vi "累积剂量查询模块.vi"() -> ()   [LabVIEW 2017]
uses:
  <vilib>/Utility/miscctls.llb/LVRowAndColumnTypeDef.ctl
  <vilib>/Utility/miscctls.llb/LVRowAndColumnUnsignedTypeDef.ctl
panel:
  in  "计数标志-刷新":i32
  in  "定时器":T1
  out "定时触发VI-引用":refnum<vi>
  in  "设备列表":T2[](array[typedef])
  in  "探测器列表":i32(listbox)
  in  "自定义导出":bool
  in  "导出条件":T5
  in  "XY图赋值错误":errorcluster caption="错误输出"
  out "刷新数据库错误":errorcluster caption="error out"
  in  "查看导出":bool
  in  "菜单项-报警列表":T6
  in  "菜单项-累积列表":T7
  in  "报警单元格位置":T8 caption="单元格位置"
  in  "累积单元格位置":T8 caption="单元格位置"
  out "信号-停止":bool=TRUE
  out "信号-刷新":bool=TRUE
  in  "刷新":bool
  in  "列数-累积表":u32
  in  "列数-报警表":u32
  out "错误输出":errorcluster
  out "累积列表选中索引":i32
  out "报警列表选中索引":i32
  out "事件-报警列表选中":refnum<user-event>
  out "事件-累积列表选中":refnum<user-event>
  in  "探测器的绑定数据":T13(array[cluster])
  out "累积剂量记录":i32(listbox)
  out "报警记录":i32(listbox)
  in  "XY图":cluster{"时间":timestamp[], "测量值":dbl[]}[](graph)
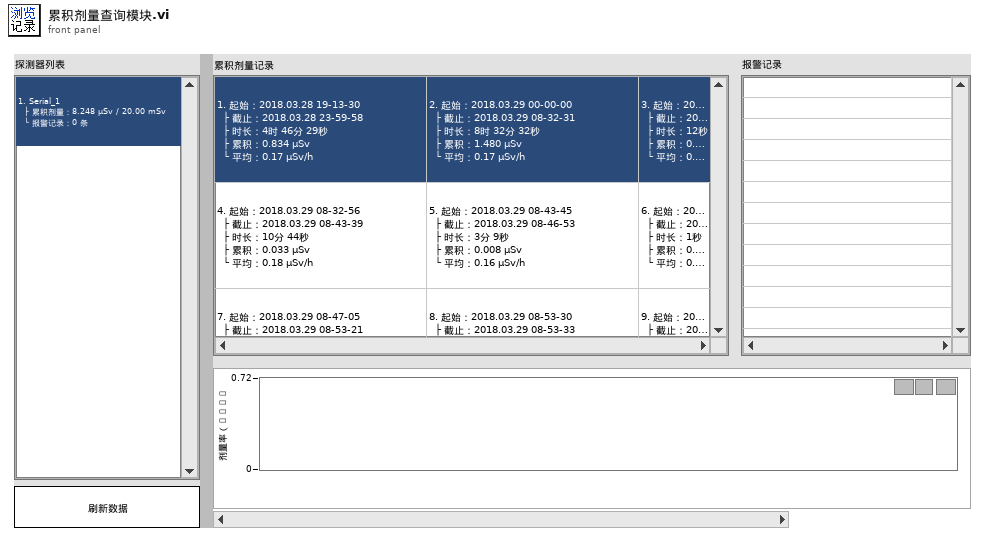
[diagram p1: front panel]
types:
  T1 = typedef "定时器枚举.ctl" = enum16{"累积定时", "导出定时"}
  T2 = typedef "探测器信息.ctl" = cluster{"网络地址":string, "名称":string, "备注":string, "累积剂量":dbl, "累积限值":dbl, "硬件剂量率限值":T3, "剂量率限值1":dbl, "剂量率限值2":dbl, "报警方式":T4}
  T3 = typedef "探头剂量率限值选择.ctl" = enum16{"一级限值", "二级限值"}
  T4 = typedef "报警方式选择.ctl" = enum16{"常报警", "自动静音", "手动静音"}
  T5 = typedef "文件导出条件.ctl" = cluster{"起始(包含)":timestamp, "截止(不含)":timestamp, "分别导出?":bool}
  T6 = typedef "菜单项-浏览界面-报警列表.ctl" = enum16{"预览"}
  T7 = typedef "菜单项-浏览界面-累积列表.ctl" = enum16{"删除选中时段"}
  T8 = typedef "LVRowAndColumnTypeDef.ctl" = cluster{"Row":i32, "Column":i32}
  T9 = typedef "单条累积记录.ctl" = cluster{"起始时间":timestamp, "结束时间":timestamp, "累积剂量":dbl}
  T10 = typedef "通用报警记录.ctl" = cluster{"探头状态":T11, "探头地址与信息":T2, "缓存绘图数据":T12, "平均值":dbl, "报警时长":cluster{"分":u16, "秒":u16}, "结论":string}
  T11 = typedef "探头状态.ctl" = enum16{"正常", "离线", "禁用", "一级报警", "二级报警", "累积报警"}
  T12 = typedef "时值缓存压缩模块.lvlib/缓存数据.ctl" = cluster{"时间":timestamp[], "数值":dbl[], "压缩等级数量":i32[], "最大值":cluster{"时间":timestamp, "数值":dbl}, "起始点":cluster{"时间":timestamp, "数值":dbl}, "容量限值":i32, "报警累积":dbl}
  T13 = cluster{"累积曲线数据":T9[], "累积列表内容":string[], "匹配的报警数据":cluster{"名称":string, "路径":path, "内容":string, "报警记录":T10}[]}[]
  T14 = typedef "浏览XY图曲线索引.ctl" = enum16{"最大值-选中", "最大值点", "率警-选中", "率警", "累积-选中", "累积-超限", "累积"}
  T15 = typedef "簇-输入.ctl" = cluster{"配置文件动作":T16, "数据输入":variant}
  T16 = typedef "枚举-配置文件动作.ctl" = enum16{"初始化加载配置", "读取配置", "写入-屏幕键盘", "写入-静音延迟", "写入-主要探头类型", "写入-串口配置", "写入-累积定时", "写入-导出定时", "保存配置到文件"}
  T17 = enum32{"Invalid", "Standard", "Closed", "Hidden", "Minimized", "Maximized"}
  T18 = typedef "簇-定时配置.ctl" = cluster{"定时模式":enum16{"绝对时间", "相对时间"}, "单位":enum16{"年", "月", "日", "时", "分"}, "间隔":u8, "目标时刻":timestamp}
  T19 = typedef "删除记录输入.ctl" = cluster{"名称":string, "多条记录(空则全删)":T9[]}
  T20 = typedef "DB动作与数据.ctl" = cluster{"动作类型":T21, "输入数据":variant}
  T21 = typedef "DB动作类型.ctl" = enum16{"DB-文件初始化+连接", "DB-断开连接", "DB-结构初始化", "DB-加载设备", "DB-检查连接状态", "设备-登记新设备+数据表", "设备-删除设备", "设备-修改网址", "设备-修改名称+转移数据", "设备-修改备注", "设备-修改限值", "设备-累积校准", "设备-重排", "数据-获取全部", "数据-删除数据", "数据-写改累积记录+改累积剂量", "读变量-全部设备"}
  T22 = typedef "簇-配置文件内容.ctl" = cluster{"调试模式？":bool, "屏幕键盘？":bool, "软件版本":string, "静音延迟 s":u16, "主要探头类型":T23, "串口配置":cluster{"COM口":refnum<visa-resource-name>, "波特率":enum16{"9600", "19200"}, "读写超时ms":i16, "丢包判定次数":i16}, "定时配置-累积分段":T18, "定时配置-自动导出":cluster{"定时配置-自动导出":T18, "分别导出?":bool}}
  T23 = typedef "枚举-主要探头类型.ctl" = enum16{"网络探头", "串口探头"}
  T24 = typedef "LVRowAndColumnUnsignedTypeDef.ctl" = cluster{"Row":u32, "Column":u32}
  T25 = cluster{"累积曲线数据":T9[], "累积列表内容":string[], "匹配的报警数据":cluster{"名称":string, "路径":path, "内容":string, "报警记录":T10}[]}
  T26 = cluster{"Shift":bool, "Ctrl":bool, "Alt":bool, "Cmd":bool, "Opt":bool}
  T27 = typedef "LVPoint32TypeDef.ctl" = cluster{"Horizontal":i32, "Vertical":i32}
  T28 = typedef "改动项选择.ctl" = enum16{"未改动", "改动-启用状态", "改动-探头信息", "改动-报警限值", "动作-手动静音", "动作-重启累积时段", "动作-累积删除", "动作-重连"}
  T29 = typedef "改动项.ctl" = cluster{"改动项选择":T28, "启用？":bool, "探测器信息":T2}
  T30 = typedef "探头属性.ctl" = cluster{"探头地址与信息":T2, "测量值":T31, "限值":T32, "探头状态":T11, "累积记录":T9, "报警方式":T33}
  T31 = typedef "测量值.ctl" = cluster{"时间":timestamp, "数值":dbl}
  T32 = typedef "剂量率限值.ctl" = cluster{"限值1":dbl, "限值2":dbl, "探头限值":T3}
  T33 = typedef "报警方式.ctl" = cluster{"报警方式":T4, "延迟计时":u16, "报警中？":bool}
  T34 = cluster{"名称":string, "路径":path, "内容":string, "报警记录":T10}[]
  T35 = cluster{"名称":string, "路径":path, "内容":string, "报警记录":T10}
  T36 = typedef "LVRectTypeDef.ctl" = cluster{"Left":i16, "Top":i16, "Right":i16, "Bottom":i16}
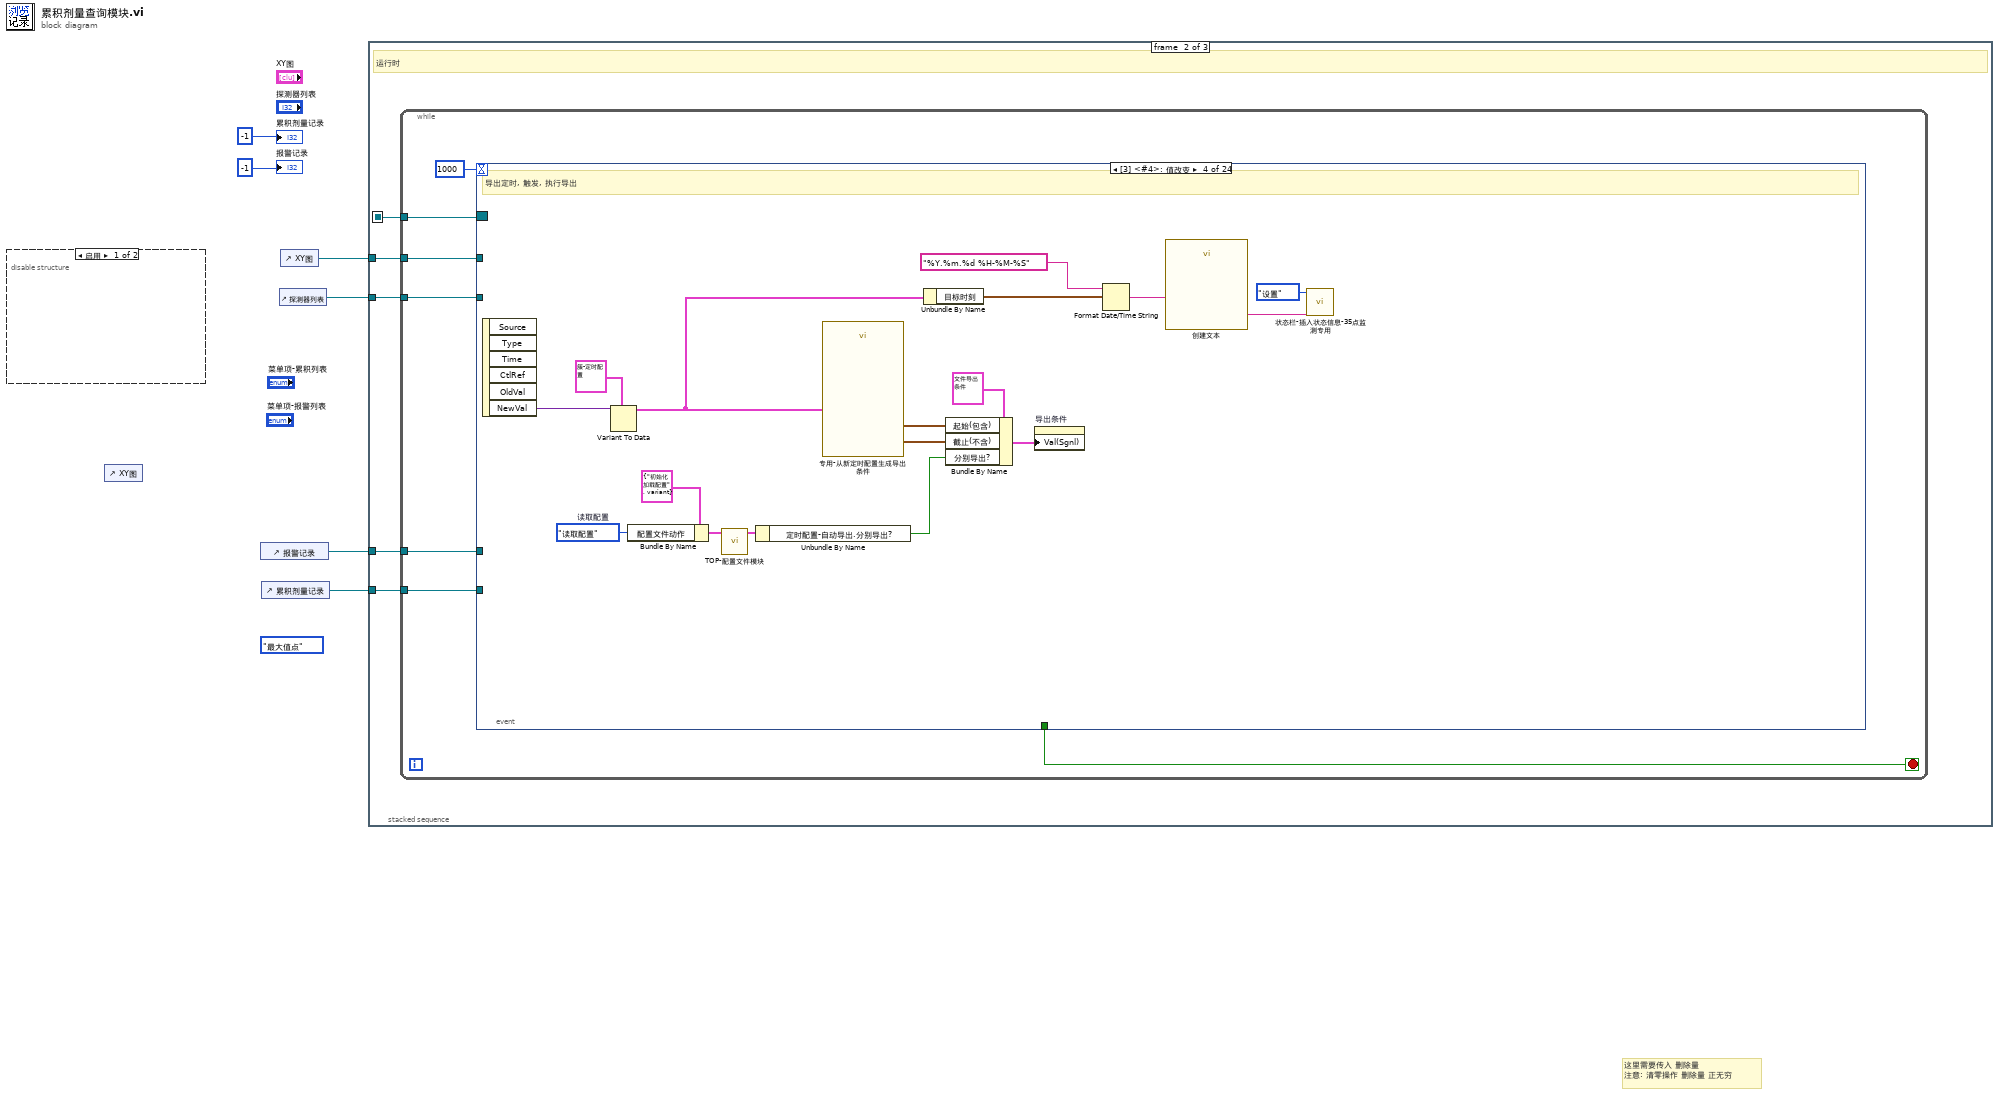
[diagram p0: block diagram]
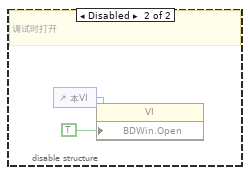
[diagram p2: hidden frame]
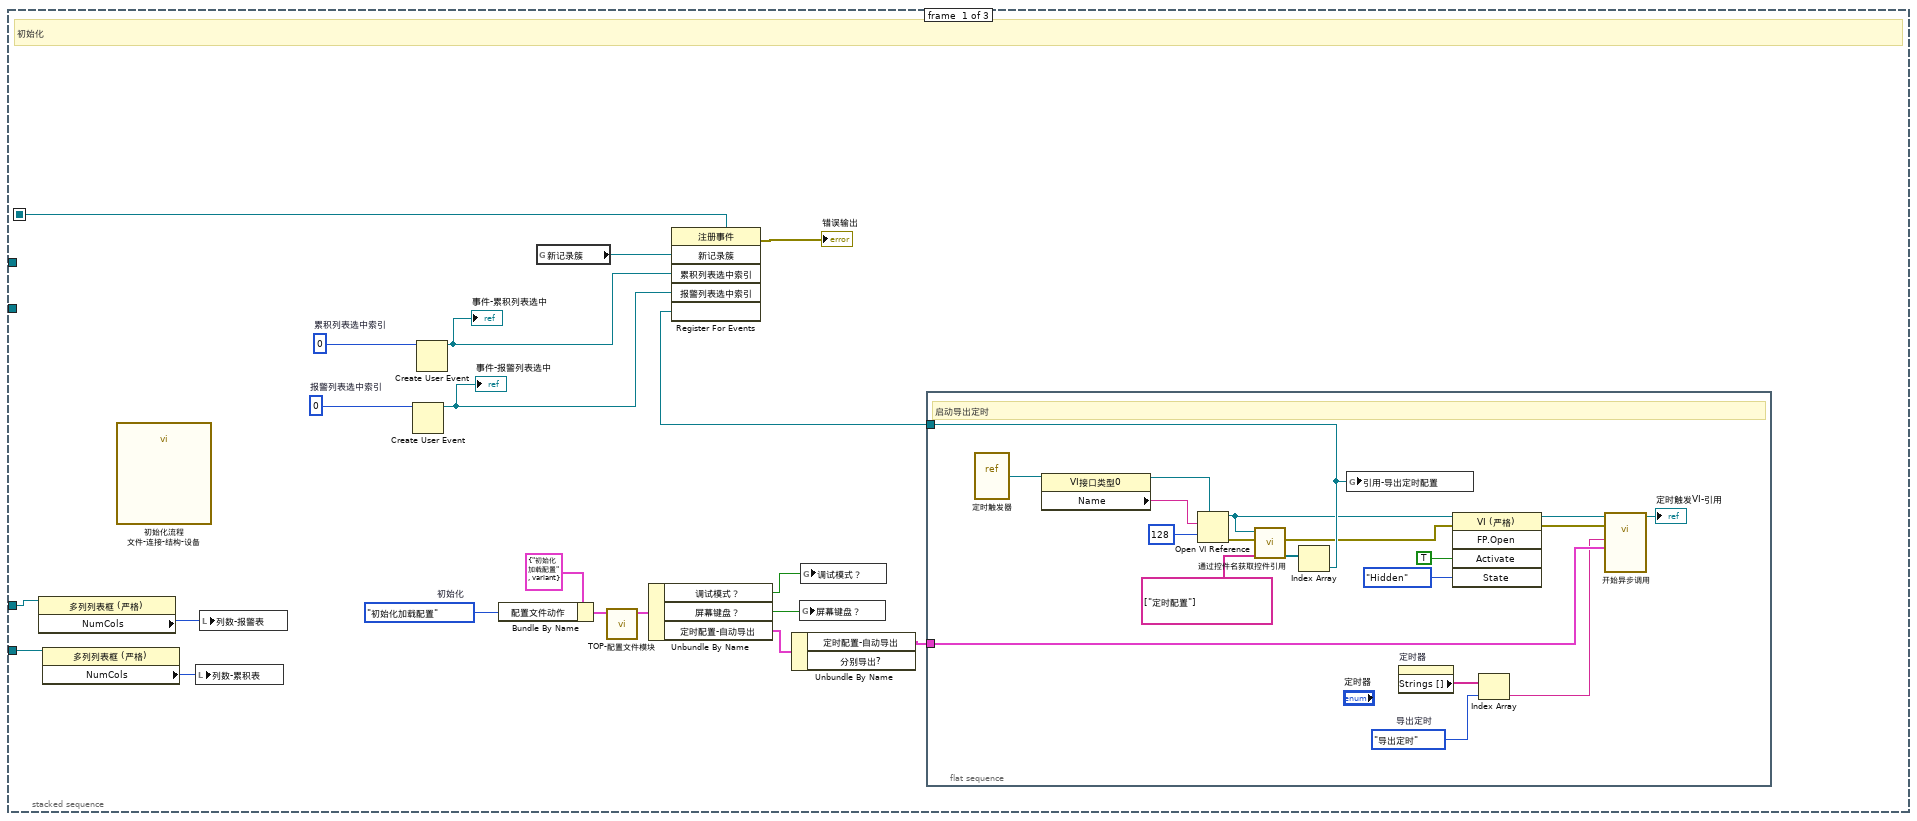
[diagram p3: hidden frame]
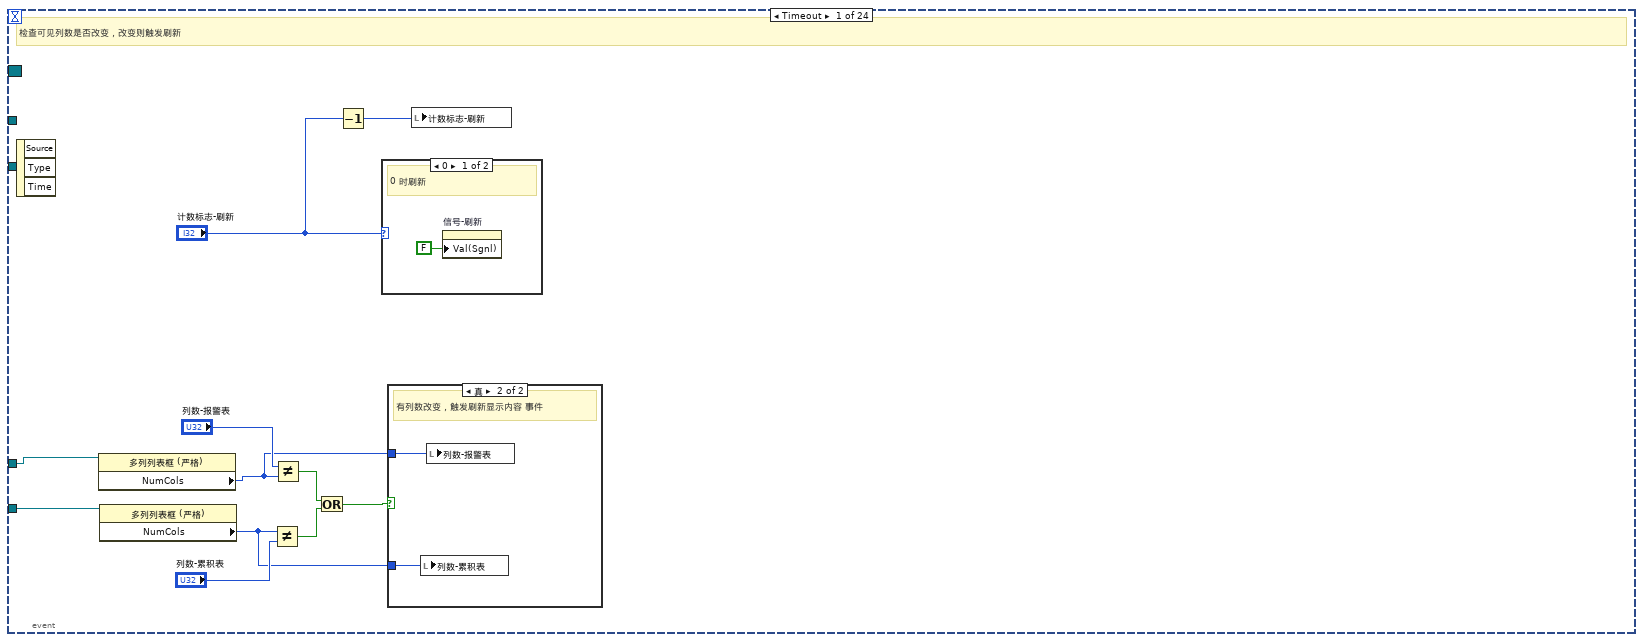
[diagram p4: hidden frame]
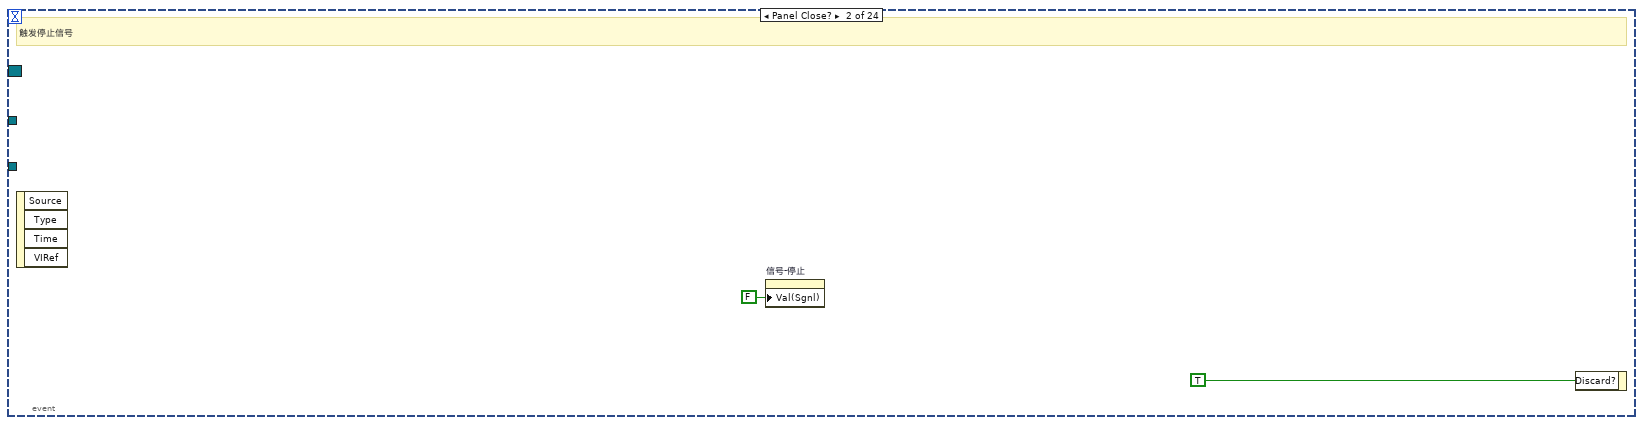
[diagram p7: hidden frame]
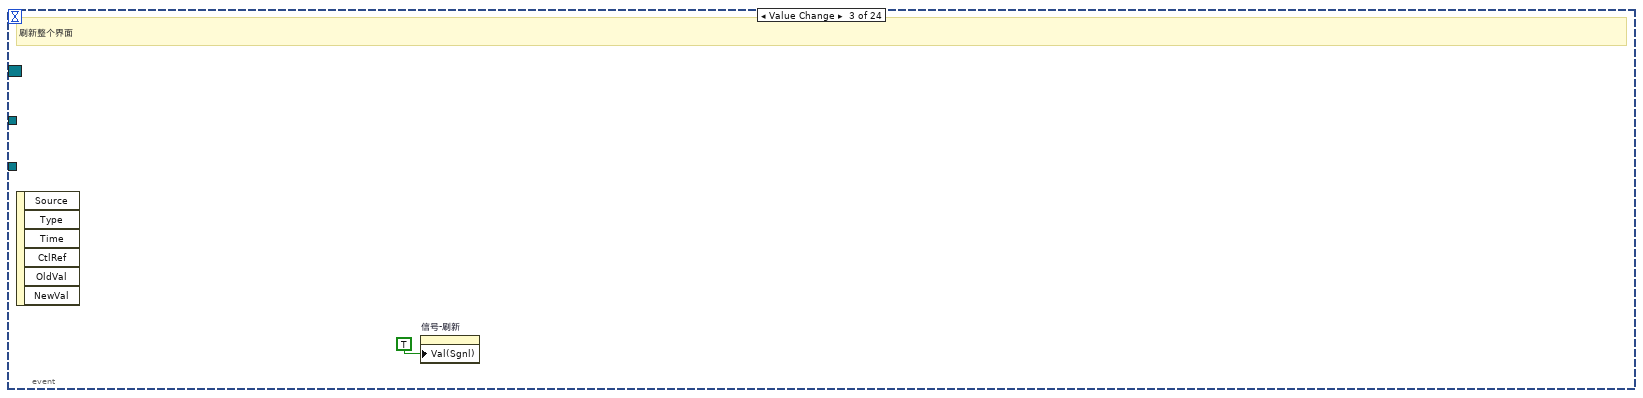
[diagram p8: hidden frame]
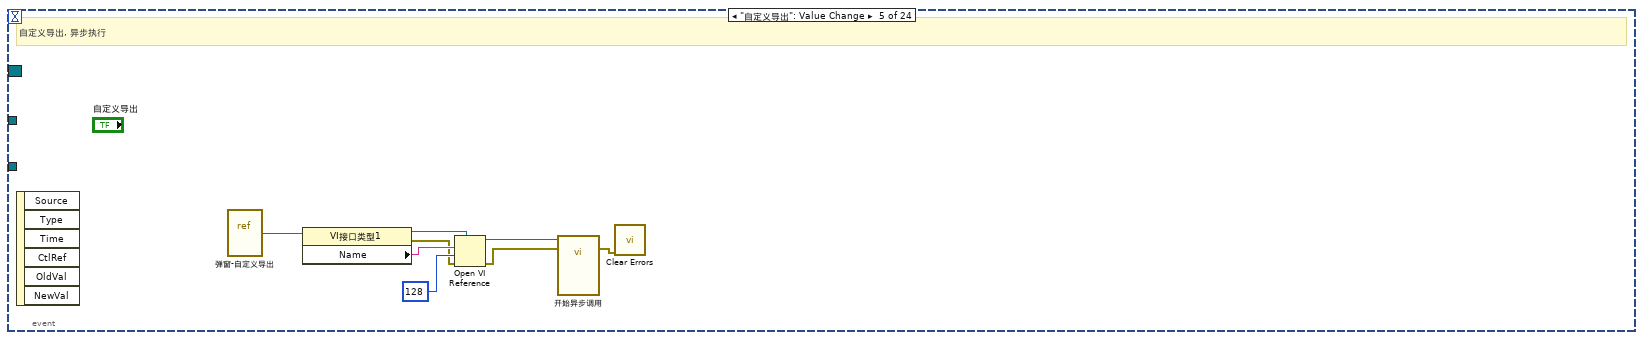
[diagram p9: hidden frame]
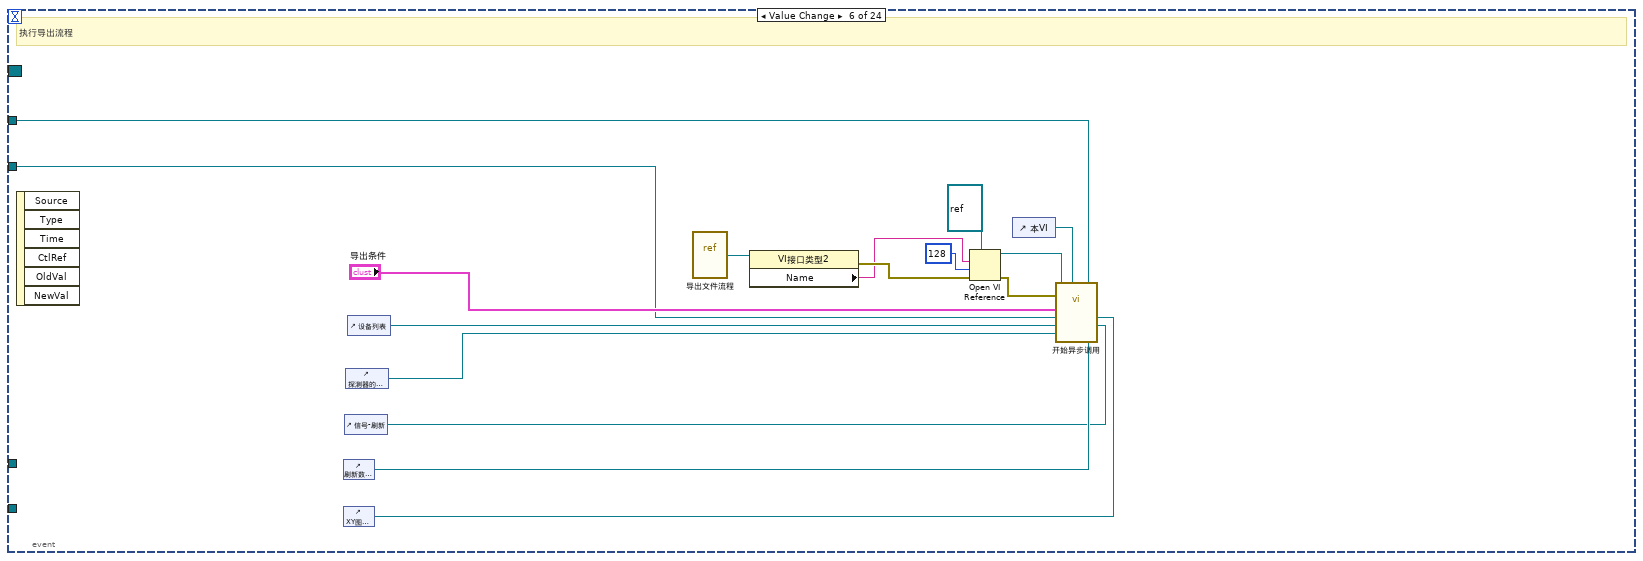
[diagram p10: hidden frame]
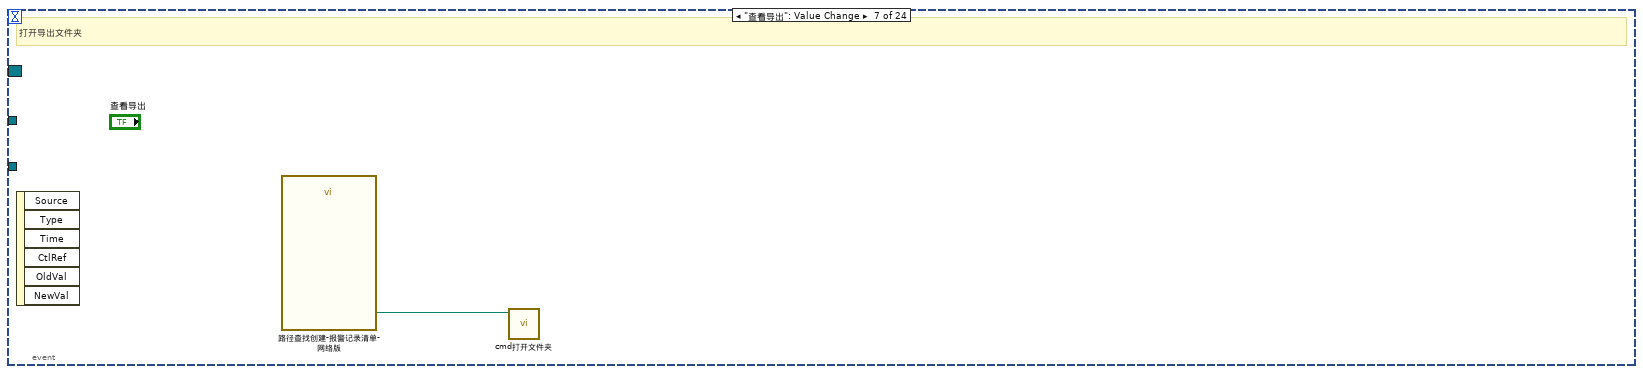
[diagram p11: hidden frame]
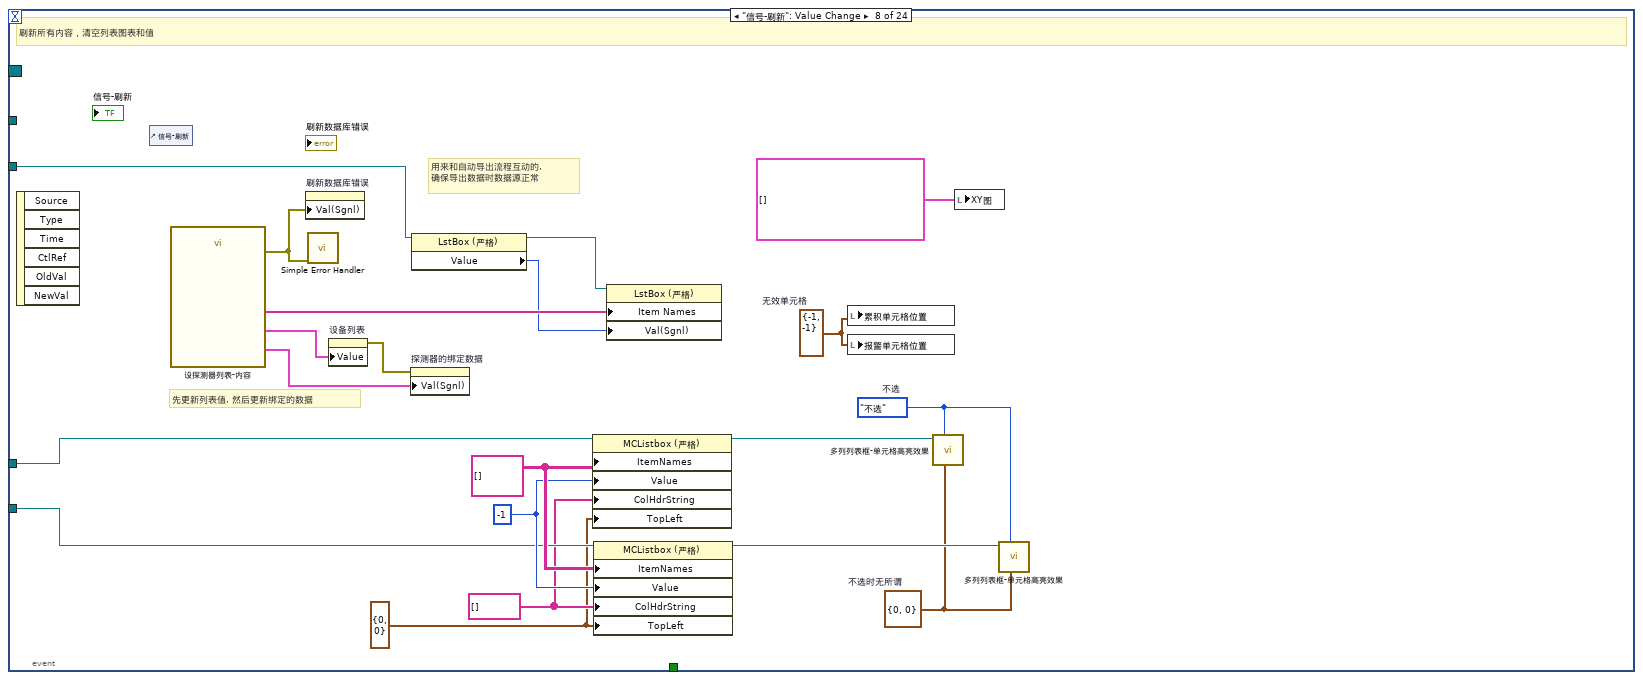
[diagram p12: hidden frame]
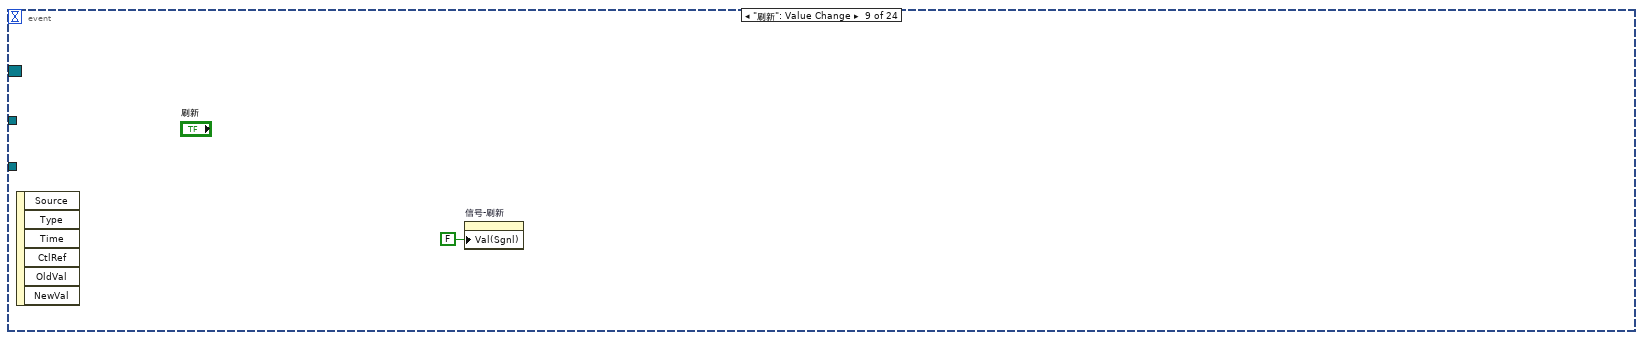
[diagram p13: hidden frame]
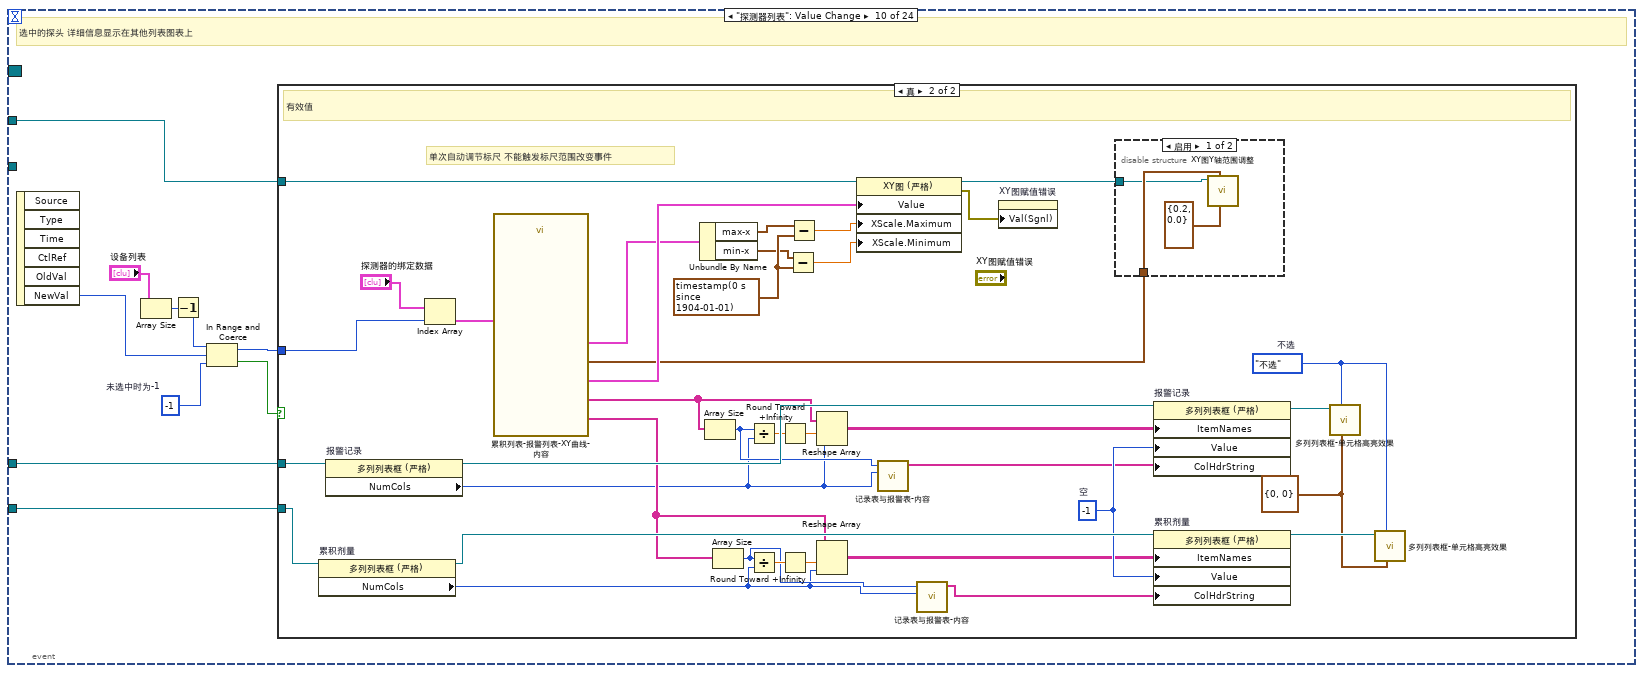
[diagram p14: hidden frame]
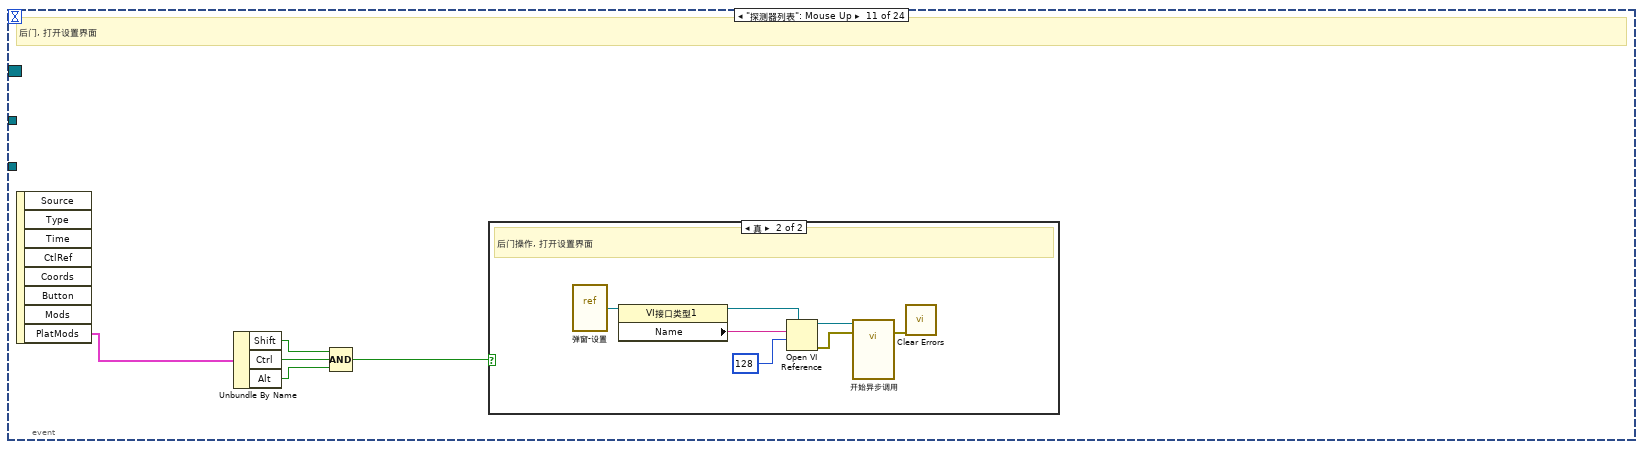
[diagram p17: hidden frame]
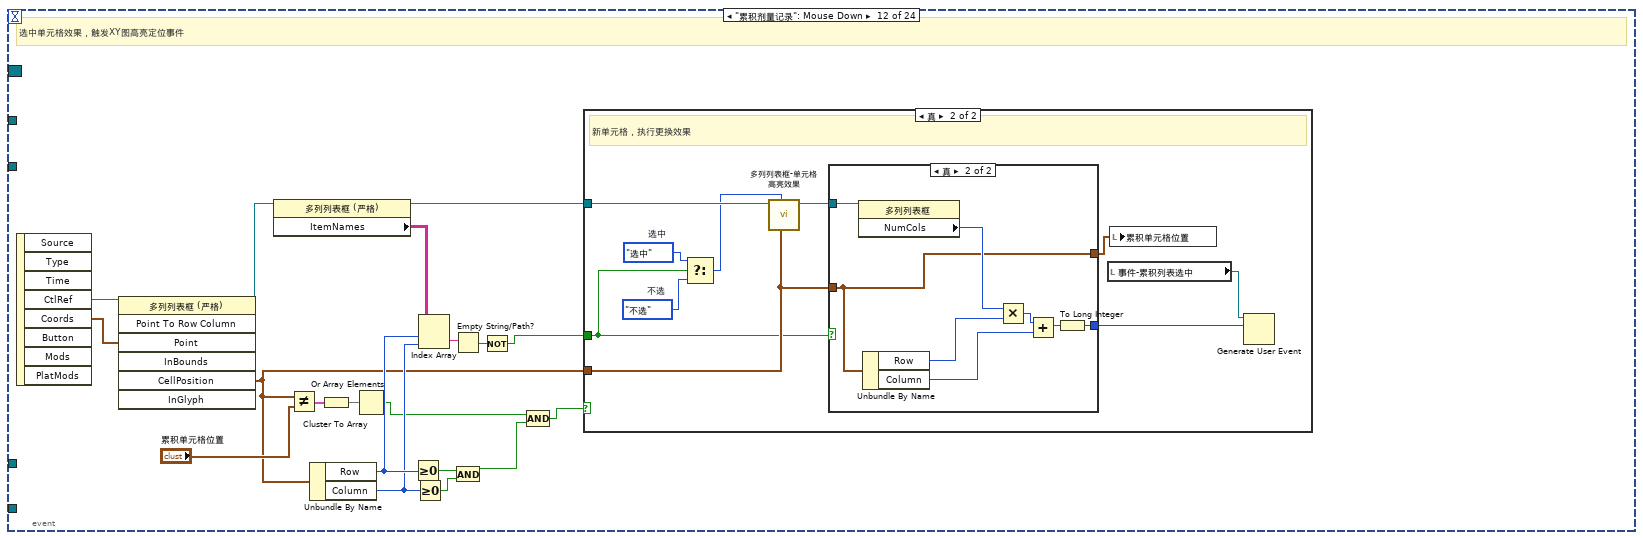
[diagram p19: hidden frame]
diagram:
  (unwired) 浏览XY图曲线索引."最大值点"
  # "这里需要传入 删除量\n注意: 清零操作 删除量 正无穷"
  n1 = disable-structure shown="启用" {
    frame Enabled {
    }
    frame Disabled {
      # "调试时打开"
      n2 = control-ref of="本VI"() -> (w7:refnum<vi>)
      n3 = property class="VI"(reference=w7, "BDWin.Open"=TRUE ("程序框图窗口:打开")) -> ()  [unwired: 1 in, 2 out]
    }
  }
  n4 = control-ref of="XY图"() -> ()  [unwired: 1 out]
  n5 = control-ref of="报警记录"() -> (w5:refnum<vi>)
  n6 = control-ref of="累积剂量记录"() -> (w4:refnum<vi>)
  n7 = control-ref of="探测器列表"() -> (w6:refnum<vi>)
  n8 = control-ref of="XY图"() -> (w3:refnum<vi>)
  n9 = stacked-sequence {
    seq-local: [w27 _ _] -> [_ w52 _]
    tunnel: w6 -> [_ w51 _]
    tunnel: w5 -> [w21 w50 _]
    tunnel: w4 -> [w20 w49 _]
    tunnel: w3 -> [_ w48 _]
    frame #0 {
      w16 = 枚举-配置文件动作."初始化加载配置"  # 初始化
      w24 = 0  # 报警列表选中索引
      w26 = 0  # 累积列表选中索引
      # "初始化"
      n10 = property class="多列列表框 (严格)"(reference=w21) -> ("NumCols"=w19:u32)  [unwired: 1 in, 2 out]
      n11 = property class="多列列表框 (严格)"(reference=w20) -> ("NumCols"=w18:u32)  [unwired: 1 in, 2 out]
      n12 = call "初始化流程 文件-连接-结构-设备.vi"() -> ()  [unwired: 10 in, 2 out]
      n13 = local write "列数-累积表"(w18) -> ()
      n14 = local write "列数-报警表"(w19) -> ()
      n15 = Create User Event(user event datatype=w24) -> (user event=w23:refnum<user-event>)  [unwired: 1 in, 1 out]
      "事件-报警列表选中" <- w23
      n16 = Create User Event(user event datatype=w26) -> (user event=w25:refnum<user-event>)  [unwired: 1 in, 1 out]
      "事件-累积列表选中" <- w25
      n17 = Bundle By Name(cluster=T15 {"配置文件动作"=enum."初始化加载配置", "数据输入"=variant} ("输入"), "配置文件动作"=w16) -> (w13:T15)
      n18 = global read "全局变量-35点监测.vi" "新记录簇"() -> (w28:refnum<vi>)
      n19 = call "TOP-配置文件模块.vi"("输入"=w13) -> ("配置文件"=w14:T22)  [unwired: 9 in, 1 out]
      n20 = Unbundle By Name(w14) -> ("调试模式？"=w10:bool, "屏幕键盘？"=w9:bool, "定时配置-自动导出"=w12:cluster{"定时配置-自动导出":T18, "分别导出?":bool})
      n21 = register-events(w28, w25, w23, w17) -> (reference out=w27:refnum<event-registration>, error out=→"错误输出":errorcluster)  [unwired: 2 in]
      n22 = Unbundle By Name(w12) -> ("定时配置-自动导出"=w11:T18)  [unwired: 1 out]
      n23 = global write "全局变量-35点监测.vi" "屏幕键盘？"(w9) -> ()
      n24 = global write "全局变量-35点监测.vi" "调试模式？"(w10) -> ()
      n25 = flat-sequence {
        tunnel: w11 -> [w40]
        tunnel: [w41] -> w17
        frame #0 {
          w31 = 定时器枚举."导出定时"  # 导出定时
          # "启动导出定时"
          n26 = vi-ref "定时触发器.vi"() -> (w45:refnum<vi>)
          n27 = property class="VI接口类型0"(reference=w45) -> (reference out=w29:refnum<vi>, "Name"=w47:string)  [unwired: 1 in, 1 out]
          n28 = Open VI Reference(type specifier VI Refnum (for type only)=w29, vi path=w47, options=128 ("选项")) -> (vi reference=w39:refnum<vi>, error out=w36:errorcluster)  [unwired: 3 in]
          n29 = call "通过控件名获取控件引用.vi"("控件名数组"=string[] ["定时配置"], "错误输入（无错误）"=w36, "VI引用"=w39) -> ("控件引用输出"=w43:refnum<vi>[], "错误输出"=w37:errorcluster)  [unwired: 6 in, 1 out]
          n30 = Index Array(array=w43) -> (element=w41:refnum<vi>)  [unwired: 1 in]
          n31 = global write "全局变量-35点监测.vi" "引用-导出定时配置"(w41) -> ()
          n32 = property on="定时器" class="Enum (严格)"() -> ("Strings []"=w32:string[])  [unwired: 2 in, 2 out]
          n33 = invoke class="VI (严格)" method="FP.Open"(reference=w39, error in=w37, "Activate"=TRUE ("激活？"), "State"=T17."Hidden" ("状态")) -> (reference out=w38:refnum<vi>, error out=w35:errorcluster)  [unwired: 1 in, 3 out]
          n34 = Index Array(array=w32, index=w31) -> (element=w30:string)
          n35 = call-by-ref "开始异步调用"(reference=w38, error in=w35, "定时配置"=w40, "定时器结构名"=w30) -> (reference out=→"定时触发VI-引用":refnum<vi>)  [unwired: 10 in, 1 out]
        }
      }
    }
    frame #1 {
      # "运行时"
      n36 = while {
        tunnel: w52 -> [w58]
        tunnel: w51 -> [w57]
        tunnel: w50 -> [w56]
        tunnel: w49 -> [w55]
        tunnel: w48 -> [w54]
        stop <- w59 stop-if-true
        n37 = event shown="[3] <#4>: 值改变" {
          selector: w58 -> [_ _ _ _ _ _ _ _ _ _ _ _ _ _ _ _ _ _ _ _ _ _ _ w578]
          dyn-events: _ -> [_ _ _ _ _ _ _ _ _ _ _ _ _ _ _ _ _ _ _ _ _ _ _ _]
          timeout: 1000 -> [_ _ _ _ _ _ _ _ _ _ _ _ _ _ _ _ _ _ _ _ _ _ _ _]
          tunnel: [_ _ _ _ _ _ _ _ _ _ _ _ _ _ _ _ _ _ _ _ _ _ _ TRUE ("放弃？")] -> w59
          tunnel: w57 -> [_ _ _ _ _ w116 _ w127 _ _ _ _ _ _ _ _ _ _ _ _ _ _ _ _]
          tunnel: w56 -> [w70 _ _ _ _ _ _ w137 _ w142 _ _ _ _ _ _ _ _ _ _ _ w443 _ _]
          tunnel: w55 -> [w69 _ _ _ _ _ _ w134 _ w143 _ _ _ _ _ _ _ _ _ _ _ w442 _ _]
          tunnel: w54 -> [_ _ _ _ _ w110 _ _ _ w141 _ _ _ _ _ _ w323 w342 _ _ _ _ _ _]
          event Timeout {
            # "检查可见列数是否改变，改变则触发刷新"
            n38 = event-data() -> ()  [unwired: 1 in, 3 out]
            n39 = property class="多列列表框 (严格)"(reference=w70) -> ("NumCols"=w62:u32)  [unwired: 1 in, 2 out]
            n40 = property class="多列列表框 (严格)"(reference=w69) -> ("NumCols"=w63:u32)  [unwired: 1 in, 2 out]
            n41 = Not Equal?(x=w63, y="列数-累积表") -> (x != y?=w66:bool)
            n42 = Not Equal?(x="列数-报警表", y=w62) -> (x != y?=w65:bool)
            n43 = Or(x=w65, y=w66) -> (x .or. y?=w64:bool)
            n44 = Decrement(x="计数标志-刷新") -> (x-1=w60:i32)
            n45 = case shown="0" "计数标志-刷新" {
              frame 0 {
                # "0 时刷新"
                n46 = property on="信号-刷新" class="Bool (严格)"("Val(Sgnl)"=FALSE ("值(信号)")) -> ()  [unwired: 2 in, 2 out]
              }
              frame 1, Default {
              }
            }
            n47 = case shown="真" w64 {
              tunnel: w63 -> [_ w72]
              tunnel: w62 -> [_ w73]
              frame False {
              }
              frame True {
                # "有列数改变，触发刷新显示内容 事件"
                n48 = local write "列数-累积表"(w72) -> ()
                n49 = local write "列数-报警表"(w73) -> ()
              }
            }
            n50 = local write "计数标志-刷新"(w60) -> ()
          }
          event Panel Close? {
            # "触发停止信号"
            n51 = event-data() -> ()  [unwired: 1 in, 4 out]
            n52 = property on="信号-停止" class="Bool (严格)"("Val(Sgnl)"=FALSE ("值(信号)")) -> ()  [unwired: 2 in, 2 out]
            n53 = event-data("Discard?"=TRUE ("放弃？")) -> ()  [unwired: 1 in, 1 out]
          }
          event Value Change {
            # "刷新整个界面"
            n54 = event-data() -> ()  [unwired: 1 in, 6 out]
            n55 = property on="信号-刷新" class="Bool (严格)"("Val(Sgnl)"=TRUE ("值(信号)")) -> ()  [unwired: 2 in, 2 out]
          }
          event Value Change {
            w85 = 枚举-配置文件动作."读取配置"  # 读取配置
            # "导出定时, 触发, 执行导出"
            n56 = event-data() -> ("NewVal"=w93:variant)  [unwired: 1 in, 5 out]
            n57 = Variant To Data(type=T18 {"定时模式"=enum."绝对时间", "单位"=enum."年", "间隔"=1, "目标时刻"=timestamp(0 s since 1904-01-01)} ("定时配置"), Variant=w93) -> (data=w82:T18)  [unwired: 1 in, 1 out]
            n58 = Bundle By Name(cluster=T15 {"配置文件动作"=enum."初始化加载配置", "数据输入"=variant} ("输入"), "配置文件动作"=w85) -> (w86:T15)
            n59 = call "TOP-配置文件模块.vi"("输入"=w86) -> ("配置文件"=w84:T22)  [unwired: 9 in, 1 out]
            n60 = Unbundle By Name(w84) -> ("定时配置-自动导出.分别导出?"=w83:bool)
            n61 = call "专用-从新定时配置生成导出条件.vi"("定时配置"=w82) -> ("时间上限(不含)"=w89:timestamp, "时间下限(包含)"=w90:timestamp)  [unwired: 9 in]
            n62 = Unbundle By Name(w82) -> ("目标时刻"=w80:timestamp)
            n63 = Bundle By Name(cluster=T5 {"起始(包含)"=timestamp(0 s since 1904-01-01), "截止(不含)"=timestamp(0 s since 1904-01-01), "分别导出?"=FALSE} ("导出条件"), "起始(包含)"=w90, "截止(不含)"=w89, "分别导出?"=w83) -> (w88:T5)
            n64 = property on="导出条件" class="Clust (严格)"("Val(Sgnl)"=w88) -> ()  [unwired: 2 in, 2 out]
            n65 = Format Date/Time String(time format string (%c)="%Y.%m.%d %H-%M-%S" ("时间格式字符串(%c)"), seconds (now)=w80) -> (date/time string=w78:string)  [unwired: 1 in]
            n66 = call "创建文本"("下个_导时"=w78) -> ("Result"=w77:string)  [unwired: 13 in, 1 out]
            n67 = call "状态栏-插入状态信息-35点监测专用.vi"("消息内容"=w77, "状态类型"=enum16{"全部", "报警", "通信", "设置"}."设置") -> ()  [unwired: 10 in]
          }
          event "自定义导出": Value Change {
            # "自定义导出, 异步执行"
            n68 = event-data() -> ()  [unwired: 1 in, 6 out]
            n69 = vi-ref "弹窗-自定义导出.vi"() -> (w101:refnum<vi>)
            n70 = property class="VI接口类型1"(reference=w101) -> (reference out=w94:refnum<vi>, error out=w97:errorcluster, "Name"=w100:string)  [unwired: 1 in]
            n71 = Open VI Reference(type specifier VI Refnum (for type only)=w94, vi path=w100, options=128 ("选项"), error in (no error)=w97) -> (vi reference=w99:refnum<vi>, error out=w96:errorcluster)  [unwired: 2 in]
            n72 = call-by-ref "开始异步调用"(reference=w99, error in=w96) -> (error out=w95:errorcluster)  [unwired: 12 in, 1 out]
            n73 = call <vilib>:"Clear Errors.vi"("error in (no error)"=w95) -> ()  [unwired: 5 in, 2 out]
          }
          event Value Change {
            # "执行导出流程"
            n74 = event-data() -> ()  [unwired: 1 in, 6 out]
            n75 = control-ref of="刷新数据库错误"() -> (w113:refnum<vi>)
            n76 = control-ref of="XY图赋值错误"() -> (w111:refnum<vi>)
            n77 = control-ref of="信号-刷新"() -> (w112:refnum<vi>)
            n78 = control-ref of="探测器的绑定数据"() -> (w114:refnum<vi>)
            n79 = control-ref of="设备列表"() -> (w115:refnum<vi>)
            n80 = vi-ref "导出文件流程.vi"() -> (w109:refnum<vi>)
            n81 = property class="VI接口类型2"(reference=w109) -> (error out=w108:errorcluster, "Name"=w107:string)  [unwired: 1 in, 1 out]
            n82 = Open VI Reference(type specifier VI Refnum (for type only)=refnum<vi> refnum ("类型说明符VI引用句柄（仅用于类型）"), vi path=w107, options=128 ("选项"), error in (no error)=w108) -> (vi reference=w104:refnum<vi>, error out=w103:errorcluster)  [unwired: 2 in]
            n83 = control-ref of="本VI"() -> (w102:refnum<vi>)
            n84 = call-by-ref "开始异步调用"(reference=w104, error in=w103, "刷新错误?"=w113, "刷新信号-引用"=w112, "XY图更新错误?"=w111, "XY图-引用"=w110, "查询界面VI-引用"=w102, "累积记录-引用"=w114, "设备清单-引用"=w115, "设备列表-引用"=w116, "导出条件"="导出条件") -> ()  [unwired: 2 in, 3 out]
          }
          event "查看导出": Value Change {
            # "打开导出文件夹"
            n85 = event-data() -> ()  [unwired: 1 in, 6 out]
            n86 = call "路径查找创建-报警记录清单-网络版.vi"() -> ("导出记录"=w118:path)  [unwired: 2 in, 13 out]
            n87 = call "cmd打开文件夹.vi"("文件路径"=w118) -> ()  [unwired: 10 in, 1 out]
          }
          event "信号-刷新": Value Change {
            w119 = T24 {"Row"=0, "Column"=0} ("左上可见单元格")
            w124 = string[] [] ("项名")
            w128 = enum16{"选中", "不选"}."不选"  # 不选
            w129 = T8 {"Row"=0, "Column"=0}  # 不选时无所谓
            w130 = T8 {"Row"=-1, "Column"=-1}  # 无效单元格
            w135 = -1 ("值")
            w136 = string[][] [] ("项名")
            # "用来和自动导出流程互动的,\n确保导出数据时数据源正常"
            # "先更新列表值, 然后更新绑定的数据"
            # "刷新所有内容，清空列表图表和值"
            n88 = event-data() -> ()  [unwired: 1 in, 6 out]
            n89 = control-ref of="信号-刷新"() -> ()  [unwired: 1 out]
            n90 = call "设探测器列表-内容.vi"() -> ("error out"=w120:errorcluster, "探测器的绑定数据"=w122:T13, "探测器列表内容"=w138:string[], "设备列表"=w123:T2[])  [unwired: 8 in]
            n91 = property on="刷新数据库错误" class="Clust (严格)"("Val(Sgnl)"=w120) -> ()  [unwired: 2 in, 2 out]
            n92 = call <vilib>:"Simple Error Handler.vi"("error in (no error)"=w120) -> ()  [unwired: 4 in, 5 out]
            n93 = property on="设备列表" class="Arr (严格)"("Value"=w123) -> (error out=w121:errorcluster)  [unwired: 2 in, 1 out]
            n94 = property on="探测器的绑定数据" class="Arr (严格)"(error in=w121, "Val(Sgnl)"=w122) -> ()  [unwired: 1 in, 2 out]
            n95 = property class="LstBox (严格)"(reference=w127) -> (reference out=w126:refnum<vi>, "Value"=w125:i32)  [unwired: 1 in, 1 out]
            n96 = property class="MCListbox (严格)"(reference=w137, "ItemNames"=w136, "Value"=w135, "ColHdrString"=w124, "TopLeft"=w119) -> (reference out=w132:refnum<vi>)  [unwired: 1 in, 1 out]
            n97 = property class="MCListbox (严格)"(reference=w134, "ItemNames"=w136, "Value"=w135, "ColHdrString"=w124, "TopLeft"=w119) -> (reference out=w131:refnum<vi>)  [unwired: 1 in, 1 out]
            n98 = property class="LstBox (严格)"(reference=w126, "Item Names"=w138, "Val(Sgnl)"=w125) -> ()  [unwired: 1 in, 2 out]
            n99 = local write "累积单元格位置"(w130) -> ()
            n100 = local write "报警单元格位置"(w130) -> ()
            n101 = call "多列列表框-单元格高亮效果.vi"("活动单元格"=w129, "动作（选中）"=w128, "引用"=w132) -> ()  [unwired: 7 in, 2 out]
            n102 = local write "XY图"(cluster{"时间":timestamp[], "测量值":dbl[]}[] [] ("XY图")) -> ()
            n103 = call "多列列表框-单元格高亮效果.vi"("活动单元格"=w129, "动作（选中）"=w128, "引用"=w131) -> ()  [unwired: 7 in, 2 out]
          }
          event "刷新": Value Change {
            n104 = event-data() -> ()  [unwired: 1 in, 6 out]
            n105 = property on="信号-刷新" class="Bool (严格)"("Val(Sgnl)"=FALSE ("值(信号)")) -> ()  [unwired: 2 in, 2 out]
          }
          event "探测器列表": Value Change {
            w146 = -1  # 未选中时为-1
            # "选中的探头 详细信息显示在其他列表图表上"
            n106 = event-data() -> ("NewVal"=w149:i32)  [unwired: 1 in, 5 out]
            n107 = Array Size(array="设备列表") -> (size(s)=w148:i32)
            n108 = Decrement(x=w148) -> (x-1=w147:i32)
            n109 = In Range and Coerce(upper limit=w147, x=w149, lower limit=w146) -> (coerced(x)=w144:i32, In Range?=w145:bool)
            n110 = case shown="真" w145 {
              tunnel: w144 -> [_ w179]
              tunnel: w143 -> [_ w186]
              tunnel: w142 -> [_ w185]
              tunnel: w141 -> [_ w180]
              frame False {
              }
              frame True {
                w163 = timestamp(0 s since 1904-01-01)
                w166 = T8 {"Row"=0, "Column"=0} ("活动单元格")
                w167 = enum16{"选中", "不选"}."不选"  # 不选
                w182 = -1  # 空
                # "单次自动调节标尺 不能触发标尺范围改变事件"
                # "有效值"
                n111 = property on="累积剂量" class="多列列表框 (严格)"(reference=w186) -> (reference out=w183:refnum<vi>, "NumCols"=w153:u32)  [unwired: 1 in, 1 out]
                n112 = property on="报警记录" class="多列列表框 (严格)"(reference=w185) -> (reference out=w184:refnum<vi>, "NumCols"=w155:u32)  [unwired: 1 in, 1 out]
                n113 = Index Array(array="探测器的绑定数据", index=w179) -> (element=w178:T25)
                n114 = call "累积列表-报警列表-XY曲线-内容.vi"("绑定的数据"=w178) -> ("时间范围"=w164:cluster{"max-x":timestamp, "min-x":timestamp}, "报警列表内容"=w175:string[], "累积列表内容"=w170:string[], "XY图曲线数据"=w165:cluster{"数组":timestamp[], "数组":dbl[]}[], "数值范围"=w160:cluster{"max-y":dbl, "min-y":dbl})  [unwired: 6 in]
                n115 = Unbundle By Name(w164) -> ("max-x"=w162:timestamp, "min-x"=w161:timestamp)
                n116 = Array Size(array=w175) -> (size(s)=w156:i32)
                n117 = Array Size(array=w170) -> (size(s)=w154:i32)
                n118 = Divide(x=w156, y=w155) -> (x/y=w177:dbl)
                n119 = Divide(x=w154, y=w153) -> (x/y=w176:dbl)
                n120 = Round Toward +Infinity(x=w177) -> (ceil(x): smallest int >= x=w174:dbl)
                n121 = Round Toward +Infinity(x=w176) -> (ceil(x): smallest int >= x=w173:dbl)
                n122 = Subtract(x=w161, y=w163) -> (x-y=w157:dbl)
                n123 = Subtract(x=w162, y=w163) -> (x-y=w158:dbl)
                n124 = Reshape Array(w175, w174, w155) -> (w172:string[][])
                n125 = Reshape Array(w170, w173, w153) -> (w171:string[][])
                n126 = property class="XY图 (严格)"(reference=w180, "Value"=w165, "XScale.Maximum"=w158, "XScale.Minimum"=w157) -> (reference out=w159:refnum<vi>, error out=w150:errorcluster)  [unwired: 1 in]
                n127 = call "记录表与报警表-内容.vi"("列数"=w155, "总大小"=w156) -> ("列首"=w151:string[])  [unwired: 9 in]
                n128 = call "记录表与报警表-内容.vi"("列数"=w153, "总大小"=w154) -> ("列首"=w152:string[])  [unwired: 9 in]
                n129 = property on="XY图赋值错误" class="Clust (严格)"("Val(Sgnl)"=w150) -> ()  [unwired: 2 in, 2 out]
                n130 = disable-structure shown="启用" {
                  disable-tunnel: w160 -> [w189 _]
                  disable-tunnel: w159 -> [w188 _]
                  frame Enabled {
                    n131 = call "XY图Y轴范围调整.vi"("留白比例"=cluster{"顶白比例":dbl, "底白比例":dbl} {"顶白比例"=0.2, "底白比例"=0.0}, "最值"=w189, "XY图引用"=w188) -> ()  [unwired: 6 in, 3 out]
                  }
                  frame Disabled {
                  }
                }
                n132 = property on="报警记录" class="多列列表框 (严格)"(reference=w184, "ItemNames"=w172, "Value"=w182, "ColHdrString"=w151) -> (reference out=w169:refnum<vi>)  [unwired: 1 in, 1 out]
                n133 = property on="累积剂量" class="多列列表框 (严格)"(reference=w183, "ItemNames"=w171, "Value"=w182, "ColHdrString"=w152) -> (reference out=w168:refnum<vi>)  [unwired: 1 in, 1 out]
                n134 = call "多列列表框-单元格高亮效果.vi"("活动单元格"=w166, "动作（选中）"=w167, "引用"=w169) -> ()  [unwired: 7 in, 2 out]
                n135 = call "多列列表框-单元格高亮效果.vi"("活动单元格"=w166, "动作（选中）"=w167, "引用"=w168) -> ()  [unwired: 7 in, 2 out]
              }
            }
          }
          event "探测器列表": Mouse Up {
            # "后门, 打开设置界面"
            n136 = event-data() -> ("PlatMods"=w190:T26)  [unwired: 1 in, 7 out]
            n137 = Unbundle By Name(w190) -> ("Shift"=w193:bool, "Ctrl"=w194:bool, "Alt"=w192:bool)
            n138 = Compound Arithmetic op=AND ("复合运算")(w193, w194, w192) -> (w191:bool)
            n139 = case shown="真" w191 {
              frame False {
              }
              frame True {
                # "后门操作, 打开设置界面"
                n140 = vi-ref "弹窗-设置.vi"() -> (w201:refnum<vi>)
                n141 = property class="VI接口类型1"(reference=w201) -> (reference out=w195:refnum<vi>, "Name"=w200:string)  [unwired: 1 in, 1 out]
                n142 = Open VI Reference(type specifier VI Refnum (for type only)=w195, vi path=w200, options=128 ("选项")) -> (vi reference=w198:refnum<vi>, error out=w197:errorcluster)  [unwired: 3 in]
                n143 = call-by-ref "开始异步调用"(reference=w198, error in=w197) -> (error out=w196:errorcluster)  [unwired: 12 in, 1 out]
                n144 = call <vilib>:"Clear Errors.vi"("error in (no error)"=w196) -> ()  [unwired: 5 in, 2 out]
              }
            }
          }
          event "累积剂量记录": Mouse Down {
            # "选中单元格效果，触发XY图高亮定位事件"
            n145 = event-data() -> ("CtlRef"=w220:refnum<vi>, "Coords"=w219:T27)  [unwired: 1 in, 6 out]
            n146 = invoke on="调用节点" class="多列列表框 (严格)" method="Point To Row Column"(reference=w220, "Point"=w219) -> (reference out=w213:refnum<vi>, "CellPosition"=w204:T8)  [unwired: 5 in, 5 out]
            n147 = property class="多列列表框 (严格)"(reference=w213) -> (reference out=w212:refnum<vi>, "ItemNames"=w209:string[][])  [unwired: 1 in, 1 out]
            n148 = Not Equal?(x=w204, y="累积单元格位置") -> (x != y?=w217:cluster{"Row":bool, "Column":bool})
            n149 = Unbundle By Name(w204) -> ("Row"=w211:i32, "Column"=w210:i32)
            n150 = Cluster To Array(cluster=w217) -> (array=w218:bool[])
            n151 = Or Array Elements(Boolean array=w218) -> (logical OR=w203:bool)
            n152 = Greater Or Equal To 0?(x=w211) -> (x >= 0?=w214:bool)
            n153 = Greater Or Equal To 0?(x=w210) -> (x >= 0?=w205:bool)
            n154 = Index Array(array=w209, index (row)=w211, index (col)=w210) -> (element=w207:string)
            n155 = Empty String/Path?(string/path=w207) -> (empty?=w208:bool)
            n156 = And(x=w214, y=w205) -> (x .and. y?=w206:bool)
            n157 = Not(x=w208) -> (.not. x?=w202:bool)
            n158 = Compound Arithmetic op=AND ("复合运算")(w203, w206) -> (w215:bool)
            n159 = case shown="真" w215 {
              tunnel: w212 -> [_ w229]
              tunnel: w204 -> [_ w228]
              tunnel: w202 -> [_ w222]
              frame False {
              }
              frame True {
                w224 = enum16{"选中", "不选"}."不选"  # 不选
                w225 = enum16{"选中", "不选"}."选中"  # 选中
                # "新单元格，执行更换效果"
                n160 = Select(t=w225, s=w222, f=w224) -> (s? t:f=w223:enum16{"选中", "不选"})
                n161 = call "多列列表框-单元格高亮效果.vi"("活动单元格"=w228, "动作（选中）"=w223, "引用"=w229) -> ("引用输出"=w227:refnum<vi>)  [unwired: 7 in, 1 out]
                n162 = case shown="真" w222 {
                  tunnel: [-1 w234] -> w230
                  tunnel: w228 -> [_ w233]
                  tunnel: w227 -> [_ w238]
                  tunnel: [w231 w233] -> w221
                  frame False {
                    w231 = T8 {"Row"=-1, "Column"=-1}  # 无效单元格
                  }
                  frame True {
                    n163 = property class="多列列表框"(reference=w238) -> ("NumCols"=w237:u32)  [unwired: 1 in, 2 out]
                    n164 = Unbundle By Name(w233) -> ("Row"=w236:i32, "Column"=w235:i32)
                    n165 = Multiply(x=w237, y=w236) -> (x*y=w240:u32)
                    n166 = Add(x=w240, y=w235) -> (x+y=w239:u32)
                    n167 = To Long Integer(number=w239) -> (32bit integer=w234:i32)
                  }
                }
                n168 = local read "事件-累积列表选中"() -> (w226:refnum<user-event>)
                n169 = local write "累积单元格位置"(w221) -> ()
                n170 = Generate User Event(user event=w226, event data cluster=w230) -> ()  [unwired: 2 in, 2 out]
              }
            }
          }
          event "报警记录": Mouse Down {
            # "选中单元格效果，触发XY图高亮定位事件"
            n171 = event-data() -> ("CtlRef"=w259:refnum<vi>, "Coords"=w258:T27)  [unwired: 1 in, 6 out]
            n172 = invoke on="调用节点" class="多列列表框 (严格)" method="Point To Row Column"(reference=w259, "Point"=w258) -> (reference out=w245:refnum<vi>, "CellPosition"=w242:T8)  [unwired: 5 in, 5 out]
            n173 = property class="多列列表框 (严格)"(reference=w245) -> (reference out=w244:refnum<vi>, "ItemNames"=w243:string[][])  [unwired: 1 in, 1 out]
            n174 = Unbundle By Name(w242) -> ("Row"=w253:i32, "Column"=w252:i32)
            n175 = Not Equal?(x=w242, y="报警单元格位置") -> (x != y?=w256:cluster{"Row":bool, "Column":bool})
            n176 = Cluster To Array(cluster=w256) -> (array=w257:bool[])
            n177 = Or Array Elements(Boolean array=w257) -> (logical OR=w255:bool)
            n178 = Greater Or Equal To 0?(x=w253) -> (x >= 0?=w254:bool)
            n179 = Greater Or Equal To 0?(x=w252) -> (x >= 0?=w248:bool)
            n180 = Index Array(array=w243, index (row)=w253, index (col)=w252) -> (element=w250:string)
            n181 = Empty String/Path?(string/path=w250) -> (empty?=w251:bool)
            n182 = And(x=w254, y=w248) -> (x .and. y?=w249:bool)
            n183 = Not(x=w251) -> (.not. x?=w241:bool)
            n184 = Compound Arithmetic op=AND ("复合运算")(w255, w249) -> (w246:bool)
            n185 = case shown="真" w246 {
              tunnel: w244 -> [_ w268]
              tunnel: w242 -> [_ w266]
              tunnel: w241 -> [_ w264]
              frame False {
              }
              frame True {
                w263 = enum16{"选中", "不选"}."不选"  # 不选
                w262 = enum16{"选中", "不选"}."选中"  # 选中
                # "新单元格，执行更换效果"
                n186 = Select(t=w262, s=w264, f=w263) -> (s? t:f=w261:enum16{"选中", "不选"})
                n187 = call "多列列表框-单元格高亮效果.vi"("活动单元格"=w266, "动作（选中）"=w261, "引用"=w268) -> ("引用输出"=w267:refnum<vi>)  [unwired: 7 in, 1 out]
                n188 = case shown="假" w264 {
                  tunnel: [-1 w273] -> w269
                  tunnel: w267 -> [_ w277]
                  tunnel: w266 -> [_ w272]
                  tunnel: [w270 w272] -> w260
                  frame False {
                    w270 = T8 {"Row"=-1, "Column"=-1}  # 无效单元格
                  }
                  frame True {
                    n189 = Unbundle By Name(w272) -> ("Row"=w275:i32, "Column"=w274:i32)
                    n190 = property class="多列列表框"(reference=w277) -> ("NumCols"=w276:u32)  [unwired: 1 in, 2 out]
                    n191 = Multiply(x=w276, y=w275) -> (x*y=w279:u32)
                    n192 = Add(x=w279, y=w274) -> (x+y=w278:u32)
                    n193 = To Long Integer(number=w278) -> (32bit integer=w273:i32)
                  }
                }
                n194 = local read "事件-报警列表选中"() -> (w265:refnum<user-event>)
                n195 = local write "报警单元格位置"(w260) -> ()
                n196 = Generate User Event(user event=w265, event data cluster=w269) -> ()  [unwired: 2 in, 2 out]
              }
            }
          }
          event "探测器列表": Shortcut Menu Selection (User) {
            n197 = event-data() -> ("ItemTag"=w280:string)  [unwired: 1 in, 7 out]
            n198 = case shown="\"累积清零\"" w280 {
              frame "假", Default {
              }
              frame "累积清零" {
                # "菜单项, 删除累积记录数据"
                n199 = local read "探测器列表"() -> (w281:i32)
                n200 = Greater Or Equal To 0?(x=w281) -> (x >= 0?=w282:bool)
                n201 = case shown="真" w282 {
                  tunnel: w281 -> [_ w304]
                  frame False {
                  }
                  frame True {
                    w288 = 改动项选择."动作-累积删除"  # 累积删除
                    w287 = T29 {"改动项选择"=enum."未改动", "启用？"=FALSE, "探测器信息"={"网络地址"="", "名称"="", "备注"="", "累积剂量"=0.0, "累积限值"=0.0, "硬件剂量率限值"=enum."一级限值", "剂量率限值1"=0.0, "剂量率限值2"=0.0, "报警方式"=enum."常报警"}}  # 改动项
                    w302 = DB动作类型."数据-删除数据"  # 删除数据
                    # "这里需要传入 删除量\n注意: 清零操作 删除量 正无穷"
                    # "全局变量中, \"探头属性[]\" 和 \"通信单元-改动项[]-引用\" 索引是同步映射的, 可定位改动项"
                    n202 = global read "全局变量-35点监测.vi" "通信单元-改动项引用[]-引用"() -> (w294:refnum<vi>)
                    n203 = global read "全局变量-35点监测.vi" "引用-探头属性[]"() -> (w297:refnum<vi>)
                    n204 = local read "设备列表"() -> (w305:T2[])
                    n205 = property class="Arr (严格)"(reference=w297) -> ("Value"=w296:T30[])  [unwired: 1 in, 2 out]
                    n206 = Index Array(array=w305, index=w304) -> (element=w298:T2)
                    n207 = Unbundle By Name(w298) -> ("名称"=w295:string)
                    n208 = for {
                      tunnel: w296 -> [w311] mode=indexing
                      tunnel: w295 -> [w309]
                      tunnel: [w307] -> w292
                      i -> [w307]
                      stop <- w308 stop-if-true
                      # "匹配定位索引"
                      n209 = Unbundle By Name(w311) -> ("探头地址与信息.名称"=w310:string)
                      n210 = Equal?(x=w309, y=w310) -> (x = y?=w308:bool)
                    }
                    n211 = Bundle By Name(cluster=T19 {"名称"="", "多条记录(空则全删)"=[]}, "名称"=w295) -> (w303:T19)
                    n212 = Bundle By Name(cluster=T20 {"动作类型"=enum."DB-加载设备", "输入数据"=variant} ("DB动作集"), "动作类型"=w302, "输入数据"=w303) -> (w301:T20)
                    n213 = property class="Arr (严格)"(reference=w294) -> ("Value"=w293:refnum<vi>[])  [unwired: 1 in, 2 out]
                    n214 = call "TOP-累积剂量数据管理.vi"("DB动作集"=w301) -> ("error out"=w291:errorcluster, "输出数据"=w290:variant)  [unwired: 9 in]
                    n215 = Variant To Data(error in=w291, type=0.0, Variant=w290) -> (data=w284:dbl)  [unwired: 1 out]
                    n216 = Index Array(array=w293, index=w292) -> (element=w286:refnum<vi>)
                    n217 = Bundle By Name(cluster=w287, "改动项选择"=w288, "探测器信息.累积剂量"=w284) -> (w285:T29)
                    n218 = property class="Ctl"(reference=w286, "Value"=w285) -> (error out=w283:errorcluster)  [unwired: 1 in, 1 out]
                    n219 = flat-sequence {
                      tunnel: w283 -> [_]
                      frame #0 {
                        n220 = local write "计数标志-刷新"(2 ("计数标志-刷新")) -> ()
                      }
                    }
                  }
                }
              }
            }
          }
          event "累积剂量记录": Shortcut Menu Selection (User) {
            # "删除数据操作"
            n221 = event-data() -> ("ItemTag"=w314:string)  [unwired: 1 in, 7 out]
            n222 = property on="菜单项-累积列表" class="Enum (严格)"() -> ("Strings []"=w313:string[])  [unwired: 2 in, 2 out]
            n223 = Search 1D Array(1D array=w313, element=w314) -> (index of element=w312:i32)  [unwired: 1 in]
            n224 = property on="菜单项-累积列表" class="Enum (严格)"("Val(Sgnl)"=w312) -> ()  [unwired: 2 in, 2 out]
          }
          event "报警记录": Shortcut Menu Selection (User) {
            n225 = event-data() -> ("ItemTag"=w316:string)  [unwired: 1 in, 7 out]
            n226 = property on="菜单项-报警列表" class="Enum (严格)"() -> ("Strings []"=w317:string[])  [unwired: 2 in, 2 out]
            n227 = Search 1D Array(1D array=w317, element=w316) -> (index of element=w315:i32)  [unwired: 1 in]
            n228 = property on="菜单项-报警列表" class="Enum (严格)"("Val(Sgnl)"=w315) -> ()  [unwired: 2 in, 2 out]
          }
          event User Event {
            w321 = 浏览XY图曲线索引."累积-选中"  # 累积-选中
            # "曲线图 累积剂量选中高亮效果（不用XY图注释，有列表高亮单元格就够了）"
            n229 = event-data() -> ("累积列表选中索引"=w319:i32)  [unwired: 1 in, 4 out]
            "累积列表选中索引" <- w319
            n230 = property class="XYGraph (严格)"(reference=w323) -> (reference out=w322:refnum<vi>, "Value"=w320:cluster{"时间":timestamp[], "测量值":dbl[]}[])  [unwired: 1 in, 1 out]
            n231 = in-place {
              in-place-border: w320 -> [w327]
              in-place-border: w319 -> [w325]
              n232 = in-place-array #1(w320, w321) -> ()  [unwired: 1 out]
              n233 = Greater Or Equal To 0?(x=w325) -> (x >= 0?=w324:bool)
              n234 = case shown="真" w324 {
                tunnel: w327 -> [_ w338]
                tunnel: w325 -> [_ w334]
                tunnel: [_ w328] -> w326
                frame False {
                  # "未选中索引，空选中"
                }
                frame True {
                  w335 = 2 ("长度")
                  w337 = 浏览XY图曲线索引."累积"  # 累积
                  # "选中索引，获取选中数据"
                  n235 = Index Array(array=w338, index=w337) -> (element=w336:cluster{"时间":timestamp[], "测量值":dbl[]})
                  n236 = Multiply(x=w334, y=w335) -> (x*y=w331:i32)
                  n237 = Unbundle(w336) -> ("时间"=w333:timestamp[], "测量值"=w332:dbl[])
                  n238 = Array Subset(array=w333, index=w331, length=w335) -> (w330:timestamp[])
                  n239 = Array Subset(array=w332, index=w331, length=w335) -> (w329:dbl[])
                  n240 = Bundle(w330, w329) -> (w328:cluster{timestamp[], dbl[]})  [unwired: 1 in]
                }
              }
              n241 = in-place-array #1(w326) -> (w318:cluster{"时间":timestamp[], "测量值":dbl[]}[])  [unwired: 1 out]
            }
            n242 = property class="XYGraph (严格)"(reference=w322, "Val(Sgnl)"=w318) -> ()  [unwired: 1 in, 2 out]
          }
          event User Event {
            w339 = 浏览XY图曲线索引."最大值-选中"  # 率警-选中
            w344 = 浏览XY图曲线索引."率警-选中"  # 率警-选中
            # "曲线图 报警记录选中高亮效果（不用XY图注释，有列表高亮单元格就够了）"
            n243 = event-data() -> ("报警列表选中索引"=w341:i32)  [unwired: 1 in, 4 out]
            "报警列表选中索引" <- w341
            n244 = property class="XYGraph (严格)"(reference=w342) -> (reference out=w345:refnum<vi>, "Value"=w340:cluster{"时间":timestamp[], "测量值":dbl[]}[])  [unwired: 1 in, 1 out]
            n245 = in-place {
              in-place-border: w340 -> [w349]
              in-place-border: w341 -> [w347]
              n246 = in-place-array #2(w340, w344, w339) -> ()  [unwired: 2 out]
              n247 = Greater Or Equal To 0?(x=w347) -> (x >= 0?=w346:bool)
              n248 = case shown="真" w346 {
                tunnel: [_ w362] -> w350
                tunnel: w349 -> [_ w361]
                tunnel: w347 -> [_ w356]
                tunnel: [_ w351] -> w348
                frame False {
                  # "未选中 索引，空选中"
                }
                frame True {
                  w360 = 浏览XY图曲线索引."最大值点"  # 率警
                  w368 = 2 ("长度")
                  w370 = 浏览XY图曲线索引."率警"  # 率警
                  # "选中索引，获取数据"
                  n249 = Index Array(array=w361, index=w360) -> (element=w359:cluster{"时间":timestamp[], "测量值":dbl[]})
                  n250 = Index Array(array=w361, index=w370) -> (element=w369:cluster{"时间":timestamp[], "测量值":dbl[]})
                  n251 = Multiply(x=w356, y=w368) -> (x*y=w365:i32)
                  n252 = Unbundle(w359) -> ("时间"=w358:timestamp[], "测量值"=w357:dbl[])
                  n253 = Unbundle(w369) -> ("时间"=w367:timestamp[], "测量值"=w366:dbl[])
                  n254 = Index Array(array=w357, index=w356) -> (element=w354:dbl)
                  n255 = Array Subset(array=w367, index=w365, length=w368) -> (w364:timestamp[])
                  n256 = Array Subset(array=w366, index=w365, length=w368) -> (w363:dbl[])
                  n257 = Index Array(array=w358, index=w356) -> (element=w355:timestamp)
                  n258 = Bundle(w364, w363) -> (w362:cluster{timestamp[], dbl[]})  [unwired: 1 in]
                  n259 = Build Array(w354) -> (w352:dbl[])
                  n260 = Build Array(w355) -> (w353:timestamp[])
                  n261 = Bundle(w353, w352) -> (w351:cluster{timestamp[], dbl[]})  [unwired: 1 in]
                }
              }
              n262 = in-place-array #2(w350, w348) -> (w343:cluster{"时间":timestamp[], "测量值":dbl[]}[])  [unwired: 2 out]
            }
            n263 = property class="XYGraph (严格)"(reference=w345, "Val(Sgnl)"=w343) -> ()  [unwired: 1 in, 2 out]
          }
          event Value Change {
            n264 = event-data() -> ("NewVal"=w371:T7)  [unwired: 1 in, 5 out]
            n265 = case shown="\"删除选中时段\"" w371 {
              frame "删除选中时段" {
                # "从数据库中删除 选中的累积记录"
                n266 = local read "累积列表选中索引"() -> (w372:i32)
                n267 = case shown="0.." w372 {
                  selector: w372 -> [_ w390]
                  frame -1, Default {
                  }
                  frame 0.. {
                    w378 = 改动项选择."动作-累积删除"  # 累积删除
                    w377 = T29 {"改动项选择"=enum."未改动", "启用？"=FALSE, "探测器信息"={"网络地址"="", "名称"="", "备注"="", "累积剂量"=0.0, "累积限值"=0.0, "硬件剂量率限值"=enum."一级限值", "剂量率限值1"=0.0, "剂量率限值2"=0.0, "报警方式"=enum."常报警"}}  # 改动项
                    w394 = DB动作类型."数据-删除数据"  # 删除数据
                    # "输入删除量, 而不是实际值, 仅用来传递数据"
                    # "有效选中值"
                    n268 = local read "探测器的绑定数据"() -> (w399:T13)
                    n269 = global read "全局变量-35点监测.vi" "通信单元-改动项引用[]-引用"() -> (w385:refnum<vi>)
                    n270 = global read "全局变量-35点监测.vi" "引用-探头属性[]"() -> (w387:refnum<vi>)
                    n271 = local read "探测器列表"() -> (w398:i32)
                    n272 = local read "设备列表"() -> (w401:T2[])
                    n273 = Index Array(array=w399, index=w398) -> (element=w397:T25)
                    n274 = Index Array(array=w401, index=w398) -> (element=w400:T2)
                    n275 = property class="Arr (严格)"(reference=w387) -> ("Value"=w386:T30[])  [unwired: 1 in, 2 out]
                    n276 = Unbundle By Name(w397) -> ("累积曲线数据"=w391:T9[])
                    n277 = Unbundle By Name(w400) -> ("名称"=w381:string)
                    n278 = Array Subset(array=w391, index=w390, length=1 ("长度")) -> (w392:T9[])
                    n279 = for {
                      tunnel: w386 -> [w407] mode=indexing
                      tunnel: w381 -> [w405]
                      tunnel: [w403] -> w383
                      i -> [w403]
                      stop <- w404 stop-if-true
                      # "匹配定位索引"
                      n280 = Unbundle By Name(w407) -> ("探头地址与信息.名称"=w406:string)
                      n281 = Equal?(x=w405, y=w406) -> (x = y?=w404:bool)
                    }
                    n282 = Bundle By Name(cluster=T19 {"名称"="", "多条记录(空则全删)"=[]}, "名称"=w381, "多条记录(空则全删)"=w392) -> (w396:T19)
                    n283 = Bundle By Name(cluster=T20 {"动作类型"=enum."DB-文件初始化+连接", "输入数据"=variant} ("DB动作集"), "动作类型"=w394, "输入数据"=w396) -> (w393:T20)
                    n284 = property class="Arr (严格)"(reference=w385) -> ("Value"=w384:refnum<vi>[])  [unwired: 1 in, 2 out]
                    n285 = call "TOP-累积剂量数据管理.vi"("DB动作集"=w393) -> ("error out"=w373:errorcluster, "输出数据"=w374:variant)  [unwired: 9 in]
                    n286 = Index Array(array=w384, index=w383) -> (element=w382:refnum<vi>)
                    n287 = Variant To Data(error in=w373, type=0.0, Variant=w374) -> (data=w379:dbl)  [unwired: 1 out]
                    n288 = Bundle By Name(cluster=w377, "改动项选择"=w378, "探测器信息.累积剂量"=w379) -> (w376:T29)
                    n289 = property class="Ctl"(reference=w382, "Value"=w376) -> (error out=w375:errorcluster)  [unwired: 1 in, 1 out]
                    n290 = flat-sequence {
                      tunnel: w375 -> [_]
                      frame #0 {
                        n291 = local write "计数标志-刷新"(2 ("计数标志-刷新")) -> ()
                      }
                    }
                  }
                }
              }
              frame Default {
              }
            }
          }
          event Value Change {
            # "菜单项动作"
            n292 = event-data() -> ("NewVal"=w410:T6)  [unwired: 1 in, 5 out]
            n293 = local read "报警列表选中索引"() -> (w409:i32)
            n294 = case shown="0.." w409 {
              selector: w409 -> [_ w414]
              tunnel: [path "" ("路径") w412] -> w408
              frame -1, Default {
              }
              frame 0.. {
                # "有效索引"
                n295 = local read "探测器的绑定数据"() -> (w418:T13)
                n296 = local read "探测器列表"() -> (w417:i32)
                n297 = Index Array(array=w418, index=w417) -> (element=w416:T25)
                n298 = Unbundle By Name(w416) -> ("匹配的报警数据"=w415:T34)
                n299 = Index Array(array=w415, index=w414) -> (element=w413:T35)
                n300 = Unbundle By Name(w413) -> ("路径"=w412:path)
              }
            }
            n301 = case shown="\"预览\", 默认" w410 {
              tunnel: w408 -> [w419]
              frame "预览", Default {
                # "打开预览窗口"
                n302 = call "启动-报警记录预览窗口.vi"("报警数据缓存文件"=w419) -> ()  [unwired: 10 in, 1 out]
              }
            }
          }
          event "报警记录": Double Click {
            # "双击浏览报警记录"
            n303 = event-data() -> ("CtlRef"=w426:refnum<vi>, "Coords"=w425:T27)  [unwired: 1 in, 7 out]
            n304 = invoke class="多列列表框 (严格)" method="Point To Row Column"(reference=w426, "Point"=w425) -> ("CellPosition"=w424:T8)  [unwired: 5 in, 6 out]
            n305 = local read "报警单元格位置"() -> (w423:T8)
            n306 = Equal?(x=w424, y=w423) -> (x = y?=w422:cluster{"Row":bool, "Column":bool})
            n307 = Cluster To Array(cluster=w422) -> (array=w421:bool[])
            n308 = And Array Elements(Boolean array=w421) -> (logical AND=w420:bool)
            n309 = case shown="真" w420 {
              frame False {
              }
              frame True {
                # "确保这个双击的单元格有效"
                n310 = property on="菜单项-报警列表" class="Enum (严格)"("Val(Sgnl)"=菜单项-浏览界面-报警列表."预览" ("值(信号)")) -> ()  [unwired: 2 in, 2 out]
              }
            }
          }
          event "XY图": Mouse Up {
            # "根据点击位置，定位到相应的选中项，并曲线上高亮，报警记录优先判断"
            n311 = event-data() -> ("CtlRef"=w431:refnum<vi>, "Coords"=w428:T27)  [unwired: 1 in, 6 out]
            n312 = property class="XYGraph (严格)"(reference=w431) -> ("Plot Bounds"=w441:T36)  [unwired: 1 in, 2 out]
            n313 = invoke class="XY图 (严格)" method="Map Coords To XY"(reference=w431, "Coords"=w428) -> (reference out=w429:refnum<vi>, "XY"=w430:cluster{"X":dbl, "Y":dbl})  [unwired: 5 in, 5 out]
            n314 = Unbundle By Name(w428) -> ("Horizontal"=w436:i32, "Vertical"=w435:i32)
            n315 = Unbundle By Name(w441) -> ("Right"=w438:i16, "Left"=w437:i16, "Bottom"=w440:i16, "Top"=w439:i16)
            n316 = In Range and Coerce(upper limit=w440, x=w435, lower limit=w439) -> (In Range?=w433:bool)  [unwired: 1 out]
            n317 = In Range and Coerce(upper limit=w438, x=w436, lower limit=w437) -> (In Range?=w434:bool)  [unwired: 1 out]
            n318 = And(x=w434, y=w433) -> (x .and. y?=w432:bool)
            n319 = case shown="真" w432 {
              tunnel: w429 -> [_ w456]
              tunnel: w430 -> [_ w452]
              tunnel: w443 -> [_ w450]
              tunnel: w442 -> [_ w446]
              tunnel: w428 -> [_ w444]
              frame False {
              }
              frame True {
                w448 = 浏览XY图曲线索引."累积"  # 累积
                w451 = 浏览XY图曲线索引."率警"  # 率警
                w454 = 浏览XY图曲线索引."最大值点"  # 最大值点
                # "鼠标在曲线绘图区域中"
                n320 = property class="XYGraph (严格)"(reference=w456) -> (reference out=w445:refnum<vi>, "Value"=w455:cluster{"时间":timestamp[], "测量值":dbl[]}[])  [unwired: 1 in, 1 out]
                n321 = Index Array(array=w455, index #1=w454, index #2=w451, index #3=w448) -> (element #1=w453:cluster{"时间":timestamp[], "测量值":dbl[]}, element #2=w449:cluster{"时间":timestamp[], "测量值":dbl[]}, element #3=w447:cluster{"时间":timestamp[], "测量值":dbl[]})
                n322 = stacked-sequence {
                  tunnel: w453 -> [w460 _ _]
                  tunnel: w452 -> [_ w502 w528]
                  tunnel: w450 -> [w459 w497 _]
                  tunnel: w449 -> [_ w506 _]
                  tunnel: w447 -> [_ _ w529]
                  tunnel: w446 -> [_ _ w525]
                  tunnel: w445 -> [w458 _ _]
                  tunnel: w444 -> [w457 _ _]
                  frame #0 {
                    # "穷举匹配“最大值点”，匹配后高亮"
                    n323 = Unbundle By Name(w460) -> ("时间"=w465:timestamp[], "测量值"=w463:dbl[])
                    n324 = Subtract(x=w465, y=timestamp(0 s since 1904-01-01)) -> (x-y=w464:dbl[])
                    n325 = for {
                      tunnel: w464 -> [w484] mode=indexing
                      tunnel: w463 -> [w483] mode=indexing
                      tunnel: w457 -> [w491]
                      tunnel: [w486] -> w461
                      tunnel: [w485] -> w462
                      tunnel: w458 -> [w475]
                      i -> [w486]
                      stop <- w485 stop-if-true
                      w478 = 5
                      # "穷举，各个点比对，看是否在点内（点直径10像素）"
                      n326 = Bundle(w484, "测量值"=w483) -> (w482:cluster{dbl, "测量值":dbl})  [unwired: 1 in]
                      n327 = Unbundle By Name(w491) -> ("Horizontal"=w490:i32, "Vertical"=w489:i32)
                      n328 = invoke class="XY图 (严格)" method="Map XY To Coords"(reference=w475, "XY"=w482) -> ("Coords"=w481:T27)  [unwired: 5 in, 6 out]
                      n329 = Unbundle By Name(w481) -> ("Horizontal"=w480:i32, "Vertical"=w479:i32)
                      n330 = Add(x=w478, y=w480) -> (x+y=w476:i32)
                      n331 = Subtract(x=w480, y=w478) -> (x-y=w477:i32)
                      n332 = Add(x=w478, y=w479) -> (x+y=w493:i32)
                      n333 = Subtract(x=w479, y=w478) -> (x-y=w492:i32)
                      n334 = In Range and Coerce "x范围"(upper limit=w476, x=w490, lower limit=w477) -> (In Range?=w488:bool)  [unwired: 1 out]
                      n335 = In Range and Coerce "y范围"(upper limit=w493, x=w489, lower limit=w492) -> (In Range?=w487:bool)  [unwired: 1 out]
                      n336 = And "点中？"(x=w488, y=w487) -> (x .and. y?=w485:bool)
                    }
                    n337 = case shown="真" w462 {
                      tunnel: w461 -> [_ w472]
                      tunnel: w459 -> [_ w473]
                      frame False {
                        # "没有匹配"
                      }
                      frame True {
                        # "高亮效果"
                        n338 = property class="多列列表框 (严格)"(reference=w473) -> (reference out=w470:refnum<vi>, "NumCols"=w469:u32)  [unwired: 1 in, 1 out]
                        n339 = local read "事件-报警列表选中"() -> (w474:refnum<user-event>)
                        n340 = Quotient & Remainder(x=w472, y=w469) -> (x-y*floor(x/y)=w467:u32, floor(x/y)=w468:u32)
                        n341 = Bundle(w468, w467) -> (w471:cluster{u32, u32})  [unwired: 1 in]
                        n342 = Generate User Event(user event=w474, event data cluster=w472) -> ()  [unwired: 2 in, 2 out]
                        n343 = call "多列列表框-单元格高亮效果.vi"("活动单元格"=w471, "引用"=w470) -> ()  [unwired: 8 in, 2 out]
                      }
                    }
                  }
                  frame #1 {
                    w499 = 2  # 2
                    # "二分匹配“报警条区域”，匹配后高亮"
                    n344 = Unbundle By Name(w502) -> ("X"=w501:dbl)
                    n345 = Unbundle By Name(w506) -> ("时间"=w505:timestamp[])  [unwired: 1 out]
                    n346 = Subtract(x=w505, y=timestamp(0 s since 1904-01-01)) -> (x-y=w503:dbl[])
                    n347 = call "二分法-单数值插入一维数组位置输出.vi"("数值"=w501, "一维数组"=w503) -> ("错误输出"=w494:errorcluster, "插入此索引处"=w500:i32)  [unwired: 7 in, 1 out]
                    n348 = call <vilib>:"Clear Errors.vi"("error in (no error)"=w494) -> ()  [unwired: 5 in, 2 out]
                    n349 = Quotient & Remainder(x=w500, y=w499) -> (x-y*floor(x/y)=w498:i32, floor(x/y)=w496:i32)
                    n350 = Not Equal To 0? "奇数？"(x=w498) -> (x != 0?=w495:bool)
                    n351 = case shown="真" w495 {
                      tunnel: w496 -> [_ w508]
                      tunnel: w497 -> [_ w507]
                      frame False {
                        # "没有匹配"
                      }
                      frame True {
                        # "高亮效果"
                        n352 = property class="多列列表框 (严格)"(reference=w507) -> (reference out=w510:refnum<vi>, "TopLeft"=w515:T24, "NumRows"=w514:u32, "NumCols"=w516:u32)  [unwired: 1 in, 1 out]
                        n353 = local read "事件-报警列表选中"() -> (w519:refnum<user-event>)
                        n354 = Quotient & Remainder(x=w508, y=w516) -> (x-y*floor(x/y)=w517:u32, floor(x/y)=w509:u32)
                        n355 = Bundle(w509, w517) -> (w518:cluster{u32, u32})  [unwired: 1 in]
                        n356 = Unbundle By Name(w515) -> ("Row"=w512:u32)
                        n357 = call "多列列表框-单元格高亮效果.vi"("活动单元格"=w518, "引用"=w507) -> ()  [unwired: 8 in, 2 out]
                        n358 = Generate User Event(user event=w519, event data cluster=w508) -> ()  [unwired: 2 in, 2 out]
                        n359 = Add(x=w512, y=w514) -> (x+y=w513:u32)
                        n360 = In Range and Coerce(upper limit=w513, x=w509, lower limit=w512) -> (In Range?=w511:bool)  [unwired: 1 out]
                        n361 = case shown="假" w511 {
                          tunnel: w510 -> [w523 _]
                          tunnel: w509 -> [w521 _]
                          frame False {
                            # "单元格不可见, 设置"
                            n362 = Bundle(w521, "x-y*floor(x/y)"=u32 0) -> (w520:cluster{u32, "x-y*floor(x/y)":u32})  [unwired: 1 in]
                            n363 = property class="多列列表框 (严格)"(reference=w523, "TopLeft"=w520) -> ()  [unwired: 1 in, 2 out]
                          }
                          frame True {
                            # "高亮单元格可见"
                          }
                        }
                      }
                    }
                  }
                  frame #2 {
                    w531 = 2  # 2
                    # "二分匹配，“累积剂量区域”，匹配后高亮"
                    n364 = Unbundle By Name(w528) -> ("X"=w533:dbl)
                    n365 = Unbundle By Name(w529) -> ("时间"=w536:timestamp[])  [unwired: 1 out]
                    n366 = Subtract(x=w536, y=timestamp(0 s since 1904-01-01)) -> (x-y=w534:dbl[])
                    n367 = call "二分法-单数值插入一维数组位置输出.vi"("数值"=w533, "一维数组"=w534) -> ("错误输出"=w524:errorcluster, "插入此索引处"=w532:i32)  [unwired: 7 in, 1 out]
                    n368 = call <vilib>:"Clear Errors.vi"("error in (no error)"=w524) -> ()  [unwired: 5 in, 2 out]
                    n369 = Quotient & Remainder(x=w532, y=w531) -> (x-y*floor(x/y)=w530:i32, floor(x/y)=w527:i32)
                    n370 = Not Equal To 0? "奇数？"(x=w530) -> (x != 0?=w526:bool)
                    n371 = case shown="真" w526 {
                      tunnel: w527 -> [_ w549]
                      tunnel: w525 -> [_ w544]
                      frame False {
                        # "没有匹配"
                      }
                      frame True {
                        # "高亮效果"
                        n372 = property class="多列列表框 (严格)"(reference=w544) -> (reference out=w538:refnum<vi>, "TopLeft"=w543:T24, "NumRows"=w542:u32, "NumCols"=w545:u32)  [unwired: 1 in, 1 out]
                        n373 = Quotient & Remainder(x=w549, y=w545) -> (x-y*floor(x/y)=w546:u32, floor(x/y)=w537:u32)
                        n374 = local read "事件-累积列表选中"() -> (w547:refnum<user-event>)
                        n375 = Bundle(w537, w546) -> (w548:cluster{u32, u32})  [unwired: 1 in]
                        n376 = Unbundle By Name(w543) -> ("Row"=w540:u32)
                        n377 = call "多列列表框-单元格高亮效果.vi"("活动单元格"=w548, "引用"=w544) -> ()  [unwired: 8 in, 2 out]
                        n378 = Add(x=w540, y=w542) -> (x+y=w541:u32)
                        n379 = In Range and Coerce(upper limit=w541, x=w537, lower limit=w540) -> (In Range?=w539:bool)  [unwired: 1 out]
                        n380 = Generate User Event(user event=w547, event data cluster=w549) -> ()  [unwired: 2 in, 2 out]
                        n381 = case shown="假" w539 {
                          tunnel: w538 -> [w553 _]
                          tunnel: w537 -> [w551 _]
                          frame False {
                            # "单元格不可见, 设置"
                            n382 = Bundle(w551, "x-y*floor(x/y)"=u32 0) -> (w550:cluster{u32, "x-y*floor(x/y)":u32})  [unwired: 1 in]
                            n383 = property class="多列列表框 (严格)"(reference=w553, "TopLeft"=w550) -> ()  [unwired: 1 in, 2 out]
                          }
                          frame True {
                            # "高亮单元格可见"
                          }
                        }
                      }
                    }
                  }
                }
              }
            }
          }
          event "XY图": Scale Range Change {
            w569 = 浏览XY图曲线索引."累积"  # 累积
            w570 = 浏览XY图曲线索引."最大值点"  # 最大值点
            # "防止无曲线时候得到 0 卡住"
            # "调整Y轴的标尺范围，计算像素刻度系数"
            n384 = event-data() -> ("CtlRef"=w572:refnum<vi>)  [unwired: 1 in, 7 out]
            n385 = property class="XY图 (严格)"(reference=w572) -> (reference out=w559:refnum<vi>, "Value"=w571:cluster{"时间":timestamp[], "测量值":dbl[]}[])  [unwired: 1 in, 1 out]
            n386 = Index Array(array=w571, index #1=w570, index #2=w569) -> (element #1=w568:cluster{"时间":timestamp[], "测量值":dbl[]}, element #2=w567:cluster{"时间":timestamp[], "测量值":dbl[]})
            n387 = Unbundle By Name(w567) -> ("测量值"=w566:dbl[])
            n388 = Unbundle By Name(w568) -> ("测量值"=w565:dbl[])
            n389 = Array Max & Min(array=w565) -> (max value=w564:dbl)  [unwired: 3 out]
            n390 = Array Max & Min(array=w566) -> (max value=w563:dbl)  [unwired: 3 out]
            n391 = Max & Min "最大值"(x=w564, y=w563) -> (max(x,y)=w557:dbl)  [unwired: 1 out]
            n392 = Equal To 0?(x=w557) -> (x = 0?=w555:bool)
            n393 = Select(t=1.0, s=w555, f=w557) -> (s? t:f=w556:dbl)
            n394 = Divide(x=w556, y=0.8 ("Y标尺.范围:最小值")) -> (x/y=w560:dbl)
            n395 = property class="XY图 (严格)"(reference=w559, "YScale.Minimum"=0.0 ("Y标尺.范围:最小值"), "YScale.Maximum"=w560) -> (error out=w554:errorcluster)  [unwired: 1 in, 1 out]
            n396 = call <vilib>:"Clear Errors.vi"("error in (no error)"=w554) -> ()  [unwired: 5 in, 2 out]
          }
          event "信号-停止": Value Change {
            n397 = event-data() -> ()  [unwired: 1 in, 6 out]
            n398 = local read "定时触发VI-引用"() -> (w577:refnum<vi>)
            n399 = Unregister For Events(event registration refnum=w578) -> (error out=w576:errorcluster)  [unwired: 1 in]
            n400 = invoke class="VI (严格)" method="Abort VI"(reference=w577, error in=w576) -> (reference out=w575:refnum<vi>, error out=w574:errorcluster)  [unwired: 1 in, 1 out]
            n401 = invoke class="VI (严格)" method="FP.Close"(reference=w575, error in=w574) -> (error out=w573:errorcluster)  [unwired: 1 in, 2 out]
            n402 = call <vilib>:"Clear Errors.vi"("error in (no error)"=w573) -> ()  [unwired: 5 in, 2 out]
          }
        }
      }
    }
    frame #2 {
      # "结束"
    }
  }
  "累积剂量记录" <- -1 ("累积列表选中索引")
  "报警记录" <- -1 ("累积列表选中索引")
